vi "Dashboard Main.vi"() -> ()   [LabVIEW 2020]
uses:
  <vilib>/Utility/miscctls.llb/LVRectTypeDef.ctl
  <vilib>/Utility/miscctls.llb/LVRowAndColumnTypeDef.ctl
  <vilib>/event_ctls.llb/eventvkey.ctl
  <vilib>/Rock Robotics/WPI/DriverStation/WPI_DriverStationAllianceInfo.ctl
  b1c29fd4-b69e-4c47-bd92-218700034153.vi
  74f3c57e-8635-4bc1-b4f8-b214002a8360.vi
  a407d339-4daa-4cfa-a8dc-714c5dae658b.vi
  cd51690b-7cbe-44fb-a5f0-3232adb0ed53.vi
  a4e8d5d1-2ec3-4e81-be0b-60391cc68073.vi
  1b78be80-bab2-445d-a3e8-82f142a16380.vi
  9e807339-2903-4f51-8fcc-64b6a9381567.vi
  e75f20ac-3dfa-4544-8614-4803d6d17fbb.vi
  0137daef-9682-45ba-80b9-2d4fda8852b8.vi
  f6a63fab-964b-4051-8314-d4414a0a258c.vi
  90e0fe9d-42b1-4a72-a6c8-4b9d9b3a5a2a.vi
  f15e925d-3118-43e3-bf67-a1272bbf81dd.vi
  394886aa-4cdd-4740-8681-89e3e438764a.vi
  77a42c1f-99bf-4bb6-8218-45b49017f7dc.vi
  5abae45b-ab2b-4816-ba0c-2a0b218f6531.vi
  31f70c1d-3051-4c77-9544-a691198ba614.vi
  81d0db6a-d68a-45c3-b3b1-458879412541.vi
  7115eafd-0426-4044-a2c2-04b4175d5bfc.vi
  c235c188-eb56-46fb-93d3-e8acf396af31.vi
  115ba94a-0b26-47fa-ae73-5ec5bd9e502a.vi
  2422668c-951b-48e5-9bda-0f59c56d9c0d.vi
  7776664e-4af7-4b3d-b288-2266642a045e.vi
  ace04e1a-73bd-4435-b0d6-ff328b65c92e.vi
  6004ed5d-dfc4-4dad-95c1-8e371ea2b9cd.vi
  321ce103-7778-4bb1-9ecc-75a76fef05e9.vi
  d30e88cc-5e2b-4867-b271-53fc6d5cd4d7.vi
  fde90579-e212-4b8a-8145-a17c3e40bcbd.vi
  6c63589b-432e-4f9c-bacb-2063ed7bd576.vi
  b7dcf304-99f6-4f78-9d14-19aa8d9ea562.vi
  0480a820-69ef-45e6-a9f4-d7ff60c89e45.vi
  1c99237e-ea3d-4ecf-b7c2-61034db3ecd2.vi
  db817f79-2de4-4a0f-b1b3-d5e700c778e5.vi
  2e0df589-fb3d-4210-b682-2dd460d02044.vi
  7e0b6b61-ecd1-46e7-8bdd-33cde7d6a778.vi
  5b0403e5-003a-4f6e-89c5-e8c7c203eb26.vi
  f6dc994a-5b2f-4b9c-b35a-30746132b034.vi
  769dec14-fabd-470d-9aa2-970817a7097c.vi
  609bb688-569d-4125-8a50-26b015384e1e.vi
  de6d5f31-b9eb-4ae9-a598-d9fff82cebf9.vi
  24606ce8-9050-485a-8372-b08799457f70.vi
  c4f1d6a7-022d-437a-99da-c80f8ac5100c.vi
  c6e82f58-8c51-44a0-978c-3033ebe9f2a9.vi
  434a79fa-e0d6-40cd-a4b2-153fd9802099.vi
  16a0616d-4b31-4831-aeab-0be446d50f6a.vi
  0a8fe2ab-d060-4915-a9b5-d8978247e2b6.vi
  b1c29fd4-b69e-4c47-bd92-218700034153.vi/77c742ae-e671-49bb-a825-a6e8cebc9f63.vi
  74f3c57e-8635-4bc1-b4f8-b214002a8360.vi/77c742ae-e671-49bb-a825-a6e8cebc9f63.vi
  a407d339-4daa-4cfa-a8dc-714c5dae658b.vi/77c742ae-e671-49bb-a825-a6e8cebc9f63.vi
  cd51690b-7cbe-44fb-a5f0-3232adb0ed53.vi/77c742ae-e671-49bb-a825-a6e8cebc9f63.vi
  a4e8d5d1-2ec3-4e81-be0b-60391cc68073.vi/77c742ae-e671-49bb-a825-a6e8cebc9f63.vi
  1b78be80-bab2-445d-a3e8-82f142a16380.vi/77c742ae-e671-49bb-a825-a6e8cebc9f63.vi
  9e807339-2903-4f51-8fcc-64b6a9381567.vi/77c742ae-e671-49bb-a825-a6e8cebc9f63.vi
  e75f20ac-3dfa-4544-8614-4803d6d17fbb.vi/77c742ae-e671-49bb-a825-a6e8cebc9f63.vi
  0137daef-9682-45ba-80b9-2d4fda8852b8.vi/77c742ae-e671-49bb-a825-a6e8cebc9f63.vi
  f6a63fab-964b-4051-8314-d4414a0a258c.vi/77c742ae-e671-49bb-a825-a6e8cebc9f63.vi
  90e0fe9d-42b1-4a72-a6c8-4b9d9b3a5a2a.vi/77c742ae-e671-49bb-a825-a6e8cebc9f63.vi
  f15e925d-3118-43e3-bf67-a1272bbf81dd.vi/77c742ae-e671-49bb-a825-a6e8cebc9f63.vi
  394886aa-4cdd-4740-8681-89e3e438764a.vi/77c742ae-e671-49bb-a825-a6e8cebc9f63.vi
  77a42c1f-99bf-4bb6-8218-45b49017f7dc.vi/77c742ae-e671-49bb-a825-a6e8cebc9f63.vi
  5abae45b-ab2b-4816-ba0c-2a0b218f6531.vi/77c742ae-e671-49bb-a825-a6e8cebc9f63.vi
  31f70c1d-3051-4c77-9544-a691198ba614.vi/77c742ae-e671-49bb-a825-a6e8cebc9f63.vi
  81d0db6a-d68a-45c3-b3b1-458879412541.vi/77c742ae-e671-49bb-a825-a6e8cebc9f63.vi
  7115eafd-0426-4044-a2c2-04b4175d5bfc.vi/77c742ae-e671-49bb-a825-a6e8cebc9f63.vi
  c235c188-eb56-46fb-93d3-e8acf396af31.vi/77c742ae-e671-49bb-a825-a6e8cebc9f63.vi
  115ba94a-0b26-47fa-ae73-5ec5bd9e502a.vi/77c742ae-e671-49bb-a825-a6e8cebc9f63.vi
  2422668c-951b-48e5-9bda-0f59c56d9c0d.vi/77c742ae-e671-49bb-a825-a6e8cebc9f63.vi
  7776664e-4af7-4b3d-b288-2266642a045e.vi/77c742ae-e671-49bb-a825-a6e8cebc9f63.vi
  ace04e1a-73bd-4435-b0d6-ff328b65c92e.vi/77c742ae-e671-49bb-a825-a6e8cebc9f63.vi
  6004ed5d-dfc4-4dad-95c1-8e371ea2b9cd.vi/77c742ae-e671-49bb-a825-a6e8cebc9f63.vi
  321ce103-7778-4bb1-9ecc-75a76fef05e9.vi/77c742ae-e671-49bb-a825-a6e8cebc9f63.vi
  d30e88cc-5e2b-4867-b271-53fc6d5cd4d7.vi/77c742ae-e671-49bb-a825-a6e8cebc9f63.vi
  fde90579-e212-4b8a-8145-a17c3e40bcbd.vi/77c742ae-e671-49bb-a825-a6e8cebc9f63.vi
  6c63589b-432e-4f9c-bacb-2063ed7bd576.vi/77c742ae-e671-49bb-a825-a6e8cebc9f63.vi
  b7dcf304-99f6-4f78-9d14-19aa8d9ea562.vi/77c742ae-e671-49bb-a825-a6e8cebc9f63.vi
  0480a820-69ef-45e6-a9f4-d7ff60c89e45.vi/77c742ae-e671-49bb-a825-a6e8cebc9f63.vi
  1c99237e-ea3d-4ecf-b7c2-61034db3ecd2.vi/77c742ae-e671-49bb-a825-a6e8cebc9f63.vi
  db817f79-2de4-4a0f-b1b3-d5e700c778e5.vi/77c742ae-e671-49bb-a825-a6e8cebc9f63.vi
  2e0df589-fb3d-4210-b682-2dd460d02044.vi/77c742ae-e671-49bb-a825-a6e8cebc9f63.vi
  7e0b6b61-ecd1-46e7-8bdd-33cde7d6a778.vi/77c742ae-e671-49bb-a825-a6e8cebc9f63.vi
  5b0403e5-003a-4f6e-89c5-e8c7c203eb26.vi/77c742ae-e671-49bb-a825-a6e8cebc9f63.vi
  f6dc994a-5b2f-4b9c-b35a-30746132b034.vi/77c742ae-e671-49bb-a825-a6e8cebc9f63.vi
  769dec14-fabd-470d-9aa2-970817a7097c.vi/77c742ae-e671-49bb-a825-a6e8cebc9f63.vi
  609bb688-569d-4125-8a50-26b015384e1e.vi/77c742ae-e671-49bb-a825-a6e8cebc9f63.vi
  de6d5f31-b9eb-4ae9-a598-d9fff82cebf9.vi/77c742ae-e671-49bb-a825-a6e8cebc9f63.vi
  24606ce8-9050-485a-8372-b08799457f70.vi/77c742ae-e671-49bb-a825-a6e8cebc9f63.vi
  c4f1d6a7-022d-437a-99da-c80f8ac5100c.vi/77c742ae-e671-49bb-a825-a6e8cebc9f63.vi
  c6e82f58-8c51-44a0-978c-3033ebe9f2a9.vi/77c742ae-e671-49bb-a825-a6e8cebc9f63.vi
  434a79fa-e0d6-40cd-a4b2-153fd9802099.vi/77c742ae-e671-49bb-a825-a6e8cebc9f63.vi
  16a0616d-4b31-4831-aeab-0be446d50f6a.vi/77c742ae-e671-49bb-a825-a6e8cebc9f63.vi
  0a8fe2ab-d060-4915-a9b5-d8978247e2b6.vi/77c742ae-e671-49bb-a825-a6e8cebc9f63.vi
  <vilib>/Utility/xml.llb/Read From XML File(array).vi
  <vilib>/Utility/xml.llb/Write to XML File(string).vi
  <vilib>/Rock Robotics/Network Tables/NT Read Boolean.vi
  <vilib>/Rock Robotics/Network Tables/NT Write Number.vi
  <vilib>/Rock Robotics/Network Tables/NT Read Numeric Array.vi
  <vilib>/Rock Robotics/Network Tables/NT Write Boolean.vi
  <vilib>/Rock Robotics/Network Tables/NT Read String Array.vi
  <vilib>/Rock Robotics/Network Tables/NT Read Boolean Array.vi
  <vilib>/Rock Robotics/Network Tables/NT Write String.vi
  <vilib>/Rock Robotics/Network Tables/NT Write Numeric Array.vi
  <vilib>/Rock Robotics/WPI/Dashboard/WPI_DashboardLogging Global.vi
  <vilib>/Rock Robotics/Network Tables/NT Write String Array.vi
  <vilib>/vision/NI_Vision_Development_Module.lvlib
panel:
  in  "TCP":refnum<k5>
  out "Image Message":string="Timeout in Camera Communications"
  in  "Dashboard Tab":T1(tab)=enum."Setup/Auto"
  in  "CheckList":i32(listbox)
  in  "Enable_Streaming_GUI":bool=TRUE
  out "Robot_Profile_GUI":string
  out "Auto_Playbook_GUI":string
  in  "Driver Profile (1)":u16(ring) items=["N/A"]
  in  "Camera Name":string(combo)="limelight"
  in  "Camera Settings":T2={"Frame Rate"=20, "Compression"=60, "Size"=1, "DB Camera Config"=FALSE} {"Size" items=["640x480", "320x240", "160x120"]}
  in  "Select Autonomous Play":u16(ring) items=["N/A"]
  out "Master_Caution_GUI_0":bool caption="Mode_Butterfly"
  out "Robot_is_Autonomous_GUI_0":bool caption="Mode_Butterfly"
  out "Robot_Code_Version_GUI":string
  out "Auto_Suffix_GUI":string
  in  "Refresh_Auto_Play_List_GUI":bool
  in  "Auto_Delay_GUI":dbl format="%.1f"
  in  "Manual_Start_X":dbl=324.0 format="%.1f"
  out "Robot_X":dbl format="%.1f"
  out "Robot_Y":dbl format="%.1f"
  in  "Manual_Start_Y":dbl=50.0 format="%.1f"
  out "Robot_H_GUI":dbl format="%.1f"
  in  "Manual_Start_H":dbl format="%.1f"
  out "Range_To_Target_GUI":dbl format="%.1f"
  in  "Field Map":u16(ring) items=["N/A"]
  in  "Push_Robot_Start_GUI":bool
  in  "Export_Robot_Pose":bool
  in  "Clear_Robot_Pose_Display":bool
  in  "Dock_Dashboard":bool
  in  "Force_Human_Control_GUI":bool
  in  "Auto_Test_Mode_GUI":bool
  out "Angle_To_Target_GUI":dbl format="%.1f"
  out "Turret_H_GUI":dbl format="%.1f"
  in  "Disable_Fusion_While_Autonomous":bool
  in  "Disable_Fusion_While_Disabled":bool=TRUE
  in  "New_HUB_Height_Offset_GUI":dbl min=-99.0 max=99.0 step=1.0 format="%.1f"
  out "Current_HUB_Height_Offset_GUI":dbl format="%.1f"
  in  "Apply_New_HUB_Height_Offset_GUI":bool
  out "Robot Pose 1":cluster{dbl[], dbl[]}[](graph)
  out "Help Graphic":T3(plugin-control)
  out "Master_State_1_Indicator":bool
  out "Master_State_0_Indicator":bool
  out "Shooter_State_3_Indicator":bool
  out "Shooter_State_2_Indicator":bool
  out "Shooter_State_1_Indicator":bool
  out "Kicker_Overheating_GUI":bool
  out "Robot Pose 2":cluster{dbl[], dbl[]}[](graph)
  out "Shooter_Upper_Overheating_GUI":bool
  out "Intake_Motor_Failure_Left_GUI":bool
  out "Vision_Fault_GUI":bool
  out "Pressure_Leak_GUI":bool
  in  "Master_Safety_Override_1":bool
  in  "Manipulator_Help":bool
  in  "Driver_Help":bool
  in  "Error_Help":bool
  out "No_Secondary_Camera":bool
  out "Swerve_Shifter_Failure":bool
  out "Electrical_Fault_GUI":bool
  out "Diverting_Power_GUI":bool
  out "CAN_Bus_Fault_GUI":bool
  out "IMU_Failure_GUI":bool
  out "Robot_is_Autonomous_GUI_1":bool caption="Mode_Butterfly"
  out "LL_Valid":bool caption="Mode_Butterfly"
  out "Current_Balls_GUI":i32 format="%#.0f"
  out "Intake_Motor_Failure_Right_GUI":bool
  out "CARGO_Ret_Left":bool
  out "CARGO_Ret_Right":bool
  out "Intake_Intaking_GUI":bool caption="Mode_Butterfly"
  out "Shooter_Lower_Overheating_GUI":bool
  out "Auto_Error_GUI":bool
  in  "Clear_Errors_GUI":bool
  out "Swerve_Azimuth_Fault":bool
  out "Pressure_Transducer_GUI":dbl(slide) scale=0.0..115.0
  out "Pressure_Vent_GUI":bool
  out "Swerve_Overheating":bool
  out "Compressor_On_GUI":bool
  out "HUB_Ret_Right":bool
  out "HUB_Ret_Left":bool
  in  "Right":bool
  in  "Reticule":T4(ring)
  in  "Save":bool
  in  "Up":bool
  in  "Down":bool
  in  "Left":bool
  out "Master_Caution_GUI_1":bool caption="Mode_Butterfly"
  out "Battery_Critical_GUI":bool
  out "Battery_Voltage_GUI":dbl(slide) scale=11.0..13.0
  out "Field_Oriented_GUI":bool caption="Mode_Butterfly"
  out "Slow_Loop":bool
  out "Arm_Climber":bool
  out "Combined Camera Feed":T3(plugin-control)
  out "Pointed_At_Target_GUI":bool caption="Mode_Butterfly"
  out "Shooter_Ready_GUI":bool caption="Mode_Butterfly"
  out "Shooter_Firing_GUI":bool caption="Mode_Butterfly"
  out "Shooter_Spinning_GUI":bool caption="Mode_Butterfly"
  out "Climber_Climbing_GUI":bool caption="Mode_Butterfly"
  out "Range_To_Target_GUI_Small":dbl
  out "Angle_To_Target_GUI_Small":dbl
  out "Shooter_State_0_Indicator":bool
  out "Shooter_State_4_Indicator":bool
  in  "Auto_Indexing_Override_GUI":bool
  in  "Auto_Target_Override_GUI":bool
  in  "Camera_Override_GUI":bool
  in  "Field_Oriented_Override_GUI":bool
  in  "Apply_Radial_Firing_Delay_GUI":bool
  out "Selected_Radial_Firing_Delay_GUI":dbl format="%.2f"
  in  "New_Radial_Firing_Delay_GUI":dbl min=0.0 max=5.0 step=0.1 format="%.2f"
  out "Kicker_Temperature_GUI":dbl
  out "Kicker_Speed_GUI":dbl
  in  "New_Shooter_Setpoint_Angle_GUI":dbl=11.0 min=11.0 max=36.0 step=1.0 format="%.2f"
  out "Selected_Shooter_Setpoint_Angle_Value_GUI":dbl format="%.2f"
  in  "Home_Cowl_GUI":bool
  out "Indexer_Beam_Break_GUI":bool caption="Mode_Butterfly"
  out "Cowl_Limit_A_GUI":bool caption="Mode_Butterfly"
  out "Turret_Limit_B_GUI":bool caption="Mode_Butterfly"
  out "Turret_Limit_A_GUI":bool caption="Mode_Butterfly"
  out "Turret_Angle_GUI":dbl format="%.1f"
  out "Cowl_Angle_GUI":dbl format="%.2f"
  out "Shooter_Upper_Temperature_GUI":dbl
  out "Swerve_3_Drive_Velocity":dbl format="%.1f"
  out "Swerve_3_Azimuth_Position":dbl format="%.1f"
  out "Swerve_3_Drive_Temperature":dbl
  out "Swerve_0_Drive_Temperature":dbl
  out "Camera Perf":string
  out "Control_Loop_Time_GUI":u32
  in  "Calibrate_Wheels_GUI":bool
  in  "Home_Wheels_GUI":bool
  out "Swerve_0_Azimuth_Position":dbl format="%.1f"
  out "Swerve_0_Drive_Velocity":dbl format="%.1f"
  out "Swerve_1_Drive_Velocity":dbl format="%.1f"
  out "Swerve_1_Azimuth_Position":dbl format="%.1f"
  out "Swerve_1_Drive_Temperature":dbl
  out "Swerve_2_Drive_Velocity":dbl format="%.1f"
  out "Swerve_2_Azimuth_Position":dbl format="%.1f"
  out "Swerve_2_Drive_Temperature":dbl
  in  "Arm_Calibrate_Wheels_GUI":bool
  out "Master_Caution_GUI_2":bool caption="Mode_Butterfly"
  out "Shooter_Lower_Temperature_GUI":dbl
  out "Shooter_Upper_Speed_GUI":dbl
  in  "New_Shooter_Setpoint_Speed_GUI":dbl=2000.0 min=0.0 max=5700.0 step=100.0 format="%#.0f"
  in  "Actuator Testing":u16(ring) items=["N/A"]
  in  "Test_Actuator_Value_GUI":dbl step=0.1 format="%.2f"
  in  "Calibrate_Joysticks_GUI":bool
  in  "Arm_Calibrate_Joysticks":bool
  out "Robot_is_Autonomous_GUI_2":bool caption="Mode_Butterfly"
  in  "Test_Actuator_Period_GUI":dbl min=0.0 step=1.0 format="%.2f"
  out "Pose_Loop_Time_GUI":u32
  in  "Mute_Audible_Warnings":bool
  out "Combined Error String":string
  out "Swerve_0_Shifter_State":string
  out "Swerve_1_Shifter_State":string
  out "Swerve_3_Shifter_State":string
  out "Swerve_2_Shifter_State":string
  out "Swerve_Azimuth_Fault_Array":bool[](array[boolean])
  out "Selected_Shooter_Setpoint_Speed_Value_GUI":dbl
  in  "Apply_New_Shooter_Setpoint_GUI":bool
  in  "Selected_Shooter_Setpoint_Index":u16(ring) items=["N/A"]
  in  "Super_Test_Mode_GUI":bool
  out "Current_Driver_Profile_Setpoints_GUI":T5={"Strafe Deadband"=0.08, "Strafe Scaling"=2.0, "Strafe Maximum"=0.5, "Rotation Deadband"=0.15, "Rotation Scaling"=2.5, "Rotation Maximum"=0.5} {"Rotation Maximum" min=0.3 max=1.0 scale=0.3..1.0; "Rotation Scaling" min=1.0 max=4.0 scale=1.0..4.0; "Rotation Deadband" min=0.0 max=0.25 scale=0.0..0.25; "Strafe Maximum" min=0.3 max=1.0 scale=0.3..1.0; "Strafe Scaling" min=1.0 max=4.0 scale=1.0..4.0; "Strafe Deadband" min=0.0 max=0.25 scale=0.0..0.25}
  in  "New_Driver_Profile_Setpoints_GUI":T6={"Strafe Deadband"=0.08, "Strafe Scaling"=2.0, "Strafe Max"=0.5, "Rotate Deadband"=0.15, "Rotate Scaling"=2.5, "Rotate Max"=0.5} {"Rotate Max" min=0.3 max=1.0 format="%.2g"; "Rotate Scaling" min=1.0 max=4.0 format="%.2g"; "Rotate Deadband" min=0.0 max=0.25 format="%.2g"; "Strafe Max" min=0.3 max=1.0 format="%.2g"; "Strafe Scaling" min=1.0 max=4.0 format="%.2g"; "Strafe Deadband" min=0.0 max=0.25 format="%.2g"}
  in  "Apply_Driver_Profile_Setpoints_GUI":bool
  out "Current_Driver_Profile_GUI":string
  in  "Home_Turret_GUI":bool
  out "Shooter_Lower_Speed_GUI":dbl
  out "Tower_Beam_Break_GUI":bool caption="Mode_Butterfly"
  out "Color_Sensor_Reading_GUI":string
  out "Selected_Shooter_Setpoint_Ratio_Value_GUI":dbl format="%.2f"
  in  "New_Shooter_Setpoint_Ratio_GUI":dbl=1.0 min=0.0 max=3.0 step=0.1 format="%.2f"
  out "Climber_Active_Arm_Position_GUI":dbl format="%.1f"
  in  "Free_Tuning_Variable_GUI":dbl min=0.0 step=1.0 format="%.3f"
  in  "Apply_Firing_Delay_GUI":bool
  out "Selected_Firing_Delay_GUI":dbl format="%.2f"
  in  "New_Firing_Delay_GUI":dbl min=0.0 max=5.0 step=0.1 format="%.2f"
  out "Selected_Shooter_Setpoint_Turret_Value_GUI":dbl format="%.1f"
  in  "New_Shooter_Setpoint_Turret_GUI":dbl min=-145.0 max=145.0 step=1.0 format="%.1f"
  in  "Targeting_Override_GUI":dbl(slide)=1.0 min=0.0 max=2.0 step=1.0 scale=0.0..2.0
  out "Audible_Warnings_Enabled_GUI":bool
  out "Legal_Drivers_GUI":string[](array[string])
  out "Swerve_Shifter_Failure_Array":bool[](array[boolean])
  out "Swerve_Overheating_Array":bool[](array[boolean])
  out "NT Connection":bool
  out "Mode":T7(ring)=enum."Auto Disabled"
  out "Progress":T8 {"Test Progress" scale=0.0..100.0}
  out "Cmd Status":string
  in  "Execute Command":bool
  in  "Command Params":string[][](table)
  in  "Command Selection":i32(listbox)
  out "Tree":string(tree)
  out "Background":bool
  # "2022 Dashboard v4.2-stable"
  # "Robot Profile"
  # "Robot X Position (in)"
  # "Robot Y Position (in)"
  # "Auto Play Suffix"
  # "Auto Delay (s)"
  # "X (in)"
  # "Robot Heading (deg)"
  # "Autonomous Playbook Entry"
  # "Auto Test\nMode"
  # "Force\nHuman"
  # "Turret Heading (deg)"
  # "Y (in)"
  # "Range to Target (in)"
  # "H (deg)"
  # "Angle to Target (deg)"
  # "Undock Dashboard"
  # "Yes Camera Streaming"
  # "Stop Fusion While Auto"
  # "Stop Fusion While Disabled"
  # "+X"
  # "+Y"
  # "HUB Height Offset (in)"
  # "MASTER\nSTATES"
  # "OVERRIDES"
  # "Camera Override (3)"
  # "Robot-Oriented Drive Controls"
  # "BALLS"
  # "SHOOTER\nSTATES"
  # "Manual Indexing (4)"
  # "Lock Turret to Center"
  # "(2)"
  # "SAFETY\nOVERRIDE"
  # "11"
  # "13"
  # "0"
  # "115"
  # "Drivebase Subsytem"
  # "Shooter and Turret Subsystems"
  # "Driver Profile Configuration"
  # "Shooter Setpoints"
  # "Control"
  # "Pose"
  # "Module 1"
  # "Module 0"
  # "Kicker"
  # "Latency\n(ms)"
  # "Lower"
  # "Upper"
  # "Azimuth (deg)"
  # "Speed  (rpm)"
  # "Speed (rpm)"
  # "Temp (C)"
  # "Temp (C)"
  # "Super Test Mode"
  # "Variable (bleh)"
  # "Velocity (ft/s)"
  # "Speed Ratio"
  # "Cowl"
  # "Turret"
  # "Shifter State"
  # "Angle (deg)"
  # "Angle (deg)"
  # "Module 2"
  # "Module 3"
  # "Target Selection"
  # "Limit Switches"
  # "Azimuth (deg)"
  # "Turret (deg)"
  # "Temp (C)"
  # "Calibrate Turret"
  # "Calibrate Cowl"
  # "HUB"
  # "AUTO"
  # "HANG"
  # "Velocity (ft/s)"
  # "Shifter State"
  # "Amplitude"
  # "Period (s)"
  # "Tangential Shooting Delay (s)"
  # "Calibrate Wheels"
  # "Ball Handling Subsystem"
  # "Climber Subsystem"
  # "Radial Shooting Delay (s)"
  # "Beam Breaks"
  # "Active Arms"
  # "Calibrate Joysticks"
  # "Color"
  # "Position (in)"
  # "0"
  # "0.25"
  # "1"
  # "4"
  # "0.3"
  # "1"
  # "0"
  # "0.25"
  # "1"
  # "4"
  # "0.3"
  # "1"
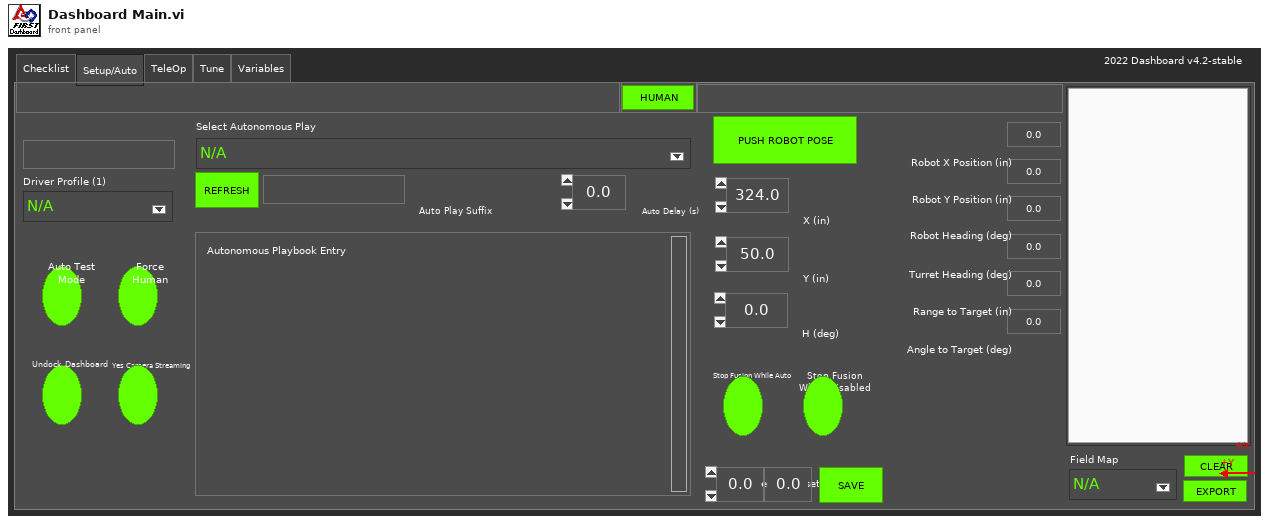
[diagram p1: front panel]
types:
  T1 = enum32{"Checklist", "Setup/Auto", "TeleOp", "Tune", "NT", "Test", "Commands", "Variables"}
  T2 = cluster{"Frame Rate":i32, "Compression":i32, "Size":u16, "DB Camera Config":bool}
  T3 = typedef "IMAQ Image.ctl" = refnum<image>
  T4 = enum16{"HUB Left Reticule", "HUB Right Reticule", "CARGO Left Reticule", "CARGO Right Reticule"}
  T5 = cluster{"Strafe Deadband":dbl, "Strafe Scaling":dbl, "Strafe Maximum":dbl, "Rotation Deadband":dbl, "Rotation Scaling":dbl, "Rotation Maximum":dbl}
  T6 = cluster{"Strafe Deadband":dbl, "Strafe Scaling":dbl, "Strafe Max":dbl, "Rotate Deadband":dbl, "Rotate Scaling":dbl, "Rotate Max":dbl}
  T7 = enum8{"Tele-Op Disabled", "Tele-Op Enabled", "Auto Disabled", "Auto Enabled", "Test Disabled", "Test Enabled", "Disconnected", "No Code", "E-Stop"}
  T8 = cluster{"Test Progress":u8, "Test Progress Text":string}
  T9 = cluster{"Save Path":path, "Interval (s)":dbl, "Keep":i32}
  T10 = enum32{"Drive", "Camera", "Basic", "Custom", "Test", "Commands", "Checklist", "Variables"}
  T11 = cluster{"IDs":cluster{"RPC field ID":u16, "Unique ID":u16}, "String":string}
  T12 = typedef "Image Type" = u32
  T13 = cluster{"HUB_Ret_Left":refnum<vi>, "HUB_Ret_Right":refnum<vi>, "CARGO_Ret_Left":refnum<vi>, "CARGO_Ret_Right":refnum<vi>}
  T14 = cluster{"Camera Name":string, string, "Saved DB Images Info":cluster{"Save Path":path, "Interval (s)":dbl, "Keep":i32}}
  T15 = typedef "WPI_DriverStationAllianceInfo.ctl" = enum16{"Red", "Blue", "Invalid"}
  T16 = enum8{"Enabled", "Disabled", "Disabled and Grayed Out"}
  T17 = cluster{"Error Strings":string, "Disable Counts":cluster{u16, u16}, "Rail Faults":cluster{u16, u16, u16}, "Robot IP":string, "DB Mode":u8, "Event Info":cluster{"Name":string, "Type":u8, "Number":u16, "Replay":u8}}
  T18 = cluster{"Storage":cluster{"Disk Free":u64, "RAM Block":u32, "RAM free":u32}, "CPU Utilization":cluster{"CPU % ISR":sgl, "CPU % Time Crit":sgl, "CPU % Timed Str":sgl, "CPU % High":sgl, "CPU % Above":sgl, "CPU % Normal":sgl, "CPU % Low":sgl}, "CAN":cluster{"% Bus Utilization":sgl, "Bus Off Cnt":u32, "TX_FIFO Full Cnt":u32, "Receive Error Cnt":u8, "Transmit Error Cnt":u8}, "HID":cluster{"HID Outputs":u32, "Rumble Low":u16, "Rumble High":u16}[]}
  T19 = cluster{"Status bits":cluster{"Test Mode":bool, "Autonomous":bool, "Enabled":bool, "Code Start":bool, "Brownout":bool, "Reserved 2":bool, "Reserved 3":bool, "E-Stop":bool}, "Code Trace":cluster{"Disabled":bool, "TeleOp":bool, "Auto":bool, "Test":bool}, "Controller Type":enum16{"unknown", "cRIO", "roboRio"}, "Code?":enum16{"unknown", "noCode", "code"}, "Battery V":dbl}
  T20 = cluster{"Control Bits":cluster{"TestMode":bool, "Autonomous":bool, "Enabled":bool, "FMS Present":bool, bool, bool, bool, "E-Stop":bool}, "Team Station ":u8, "Countdown":sgl, "Joystick Values":cluster{"Axes":dbl[], "Buttons":bool[], "POVs":i16[]}[]}
  T21 = typedef "imagedata.ctl" = cluster{"image type":i32, "image depth":i32, "image":u8[], "mask":u8[], "colors":u32[], "Rectangle":cluster{"left":i16, "top":i16, "right":i16, "bottom":i16}}
  T22 = cluster{"Boolean":bool, "Numeric Text.Text Colors:Text Color":u32}
  T23 = cluster{"Numeric Array[0]":dbl, "Numeric Array[1]":dbl, "Numeric Array[2]":dbl, "Numeric Array[3]":dbl, "Numeric Array[4]":dbl, "Numeric Array[5]":dbl}
  T24 = cluster{"Operation":enum16{"Update", "Clear"}, "Color Box":u32}[]
  T25 = typedef "eventvkey.ctl" = enum16{"ASCII", "Enter", "Return", "Shift", "Ctrl", "Alt", "Cmd", "Opt", "Caps", "NumLock", "Clear", "Break", "Up", "Down", "Left", "Right", "Insert", "Delete", "Home", "End", "PageUp", "PageDown", "Escape", "Help", "Pause", "ScrollLock", "F1", "F2", "F3", "F4", "F5", "F6", "F7", "F8", "F9", "F10", "F11", "F12", "F13", "F14", "F15", "F16", "F17", "F18", "F19", "F20", "F21", "F22", "F23", "F24", "Play", "VolumeUp", "VolumeDown", "Mute", "Two Byte Char"}
  T26 = cluster{"Operation":enum16{"Update", "Clear"}, "Color Box":u32}
  T27 = typedef "LVRowAndColumnTypeDef.ctl" = cluster{"Row":i32, "Column":i32}
  T28 = cluster{"Shift":bool, "Ctrl":bool, "Alt":bool, "Cmd":bool, "Opt":bool}
  T29 = cluster{string, "Intake_Motor_Failure_Left_GUI":bool, dbl}
  T30 = cluster{string, "Swerve_Shifter_Failure":bool, dbl}
  T31 = cluster{string, "Master_Safety_Override_1":bool, dbl}
  T32 = cluster{string, "Swerve_Azimuth_Fault":bool, dbl}
  T33 = cluster{string, "Arm_Calibrate_Wheels_GUI":bool, dbl}
  T34 = cluster{string, "Intake_Motor_Failure_Right_GUI":bool, dbl}
  T35 = cluster{string, "Electrical_Fault_GUI":bool, dbl}
  T36 = cluster{string, "Arm_Calibrate_Joysticks":bool, dbl}
  T37 = typedef "LVRectTypeDef.ctl" = cluster{"Left":i16, "Top":i16, "Right":i16, "Bottom":i16}
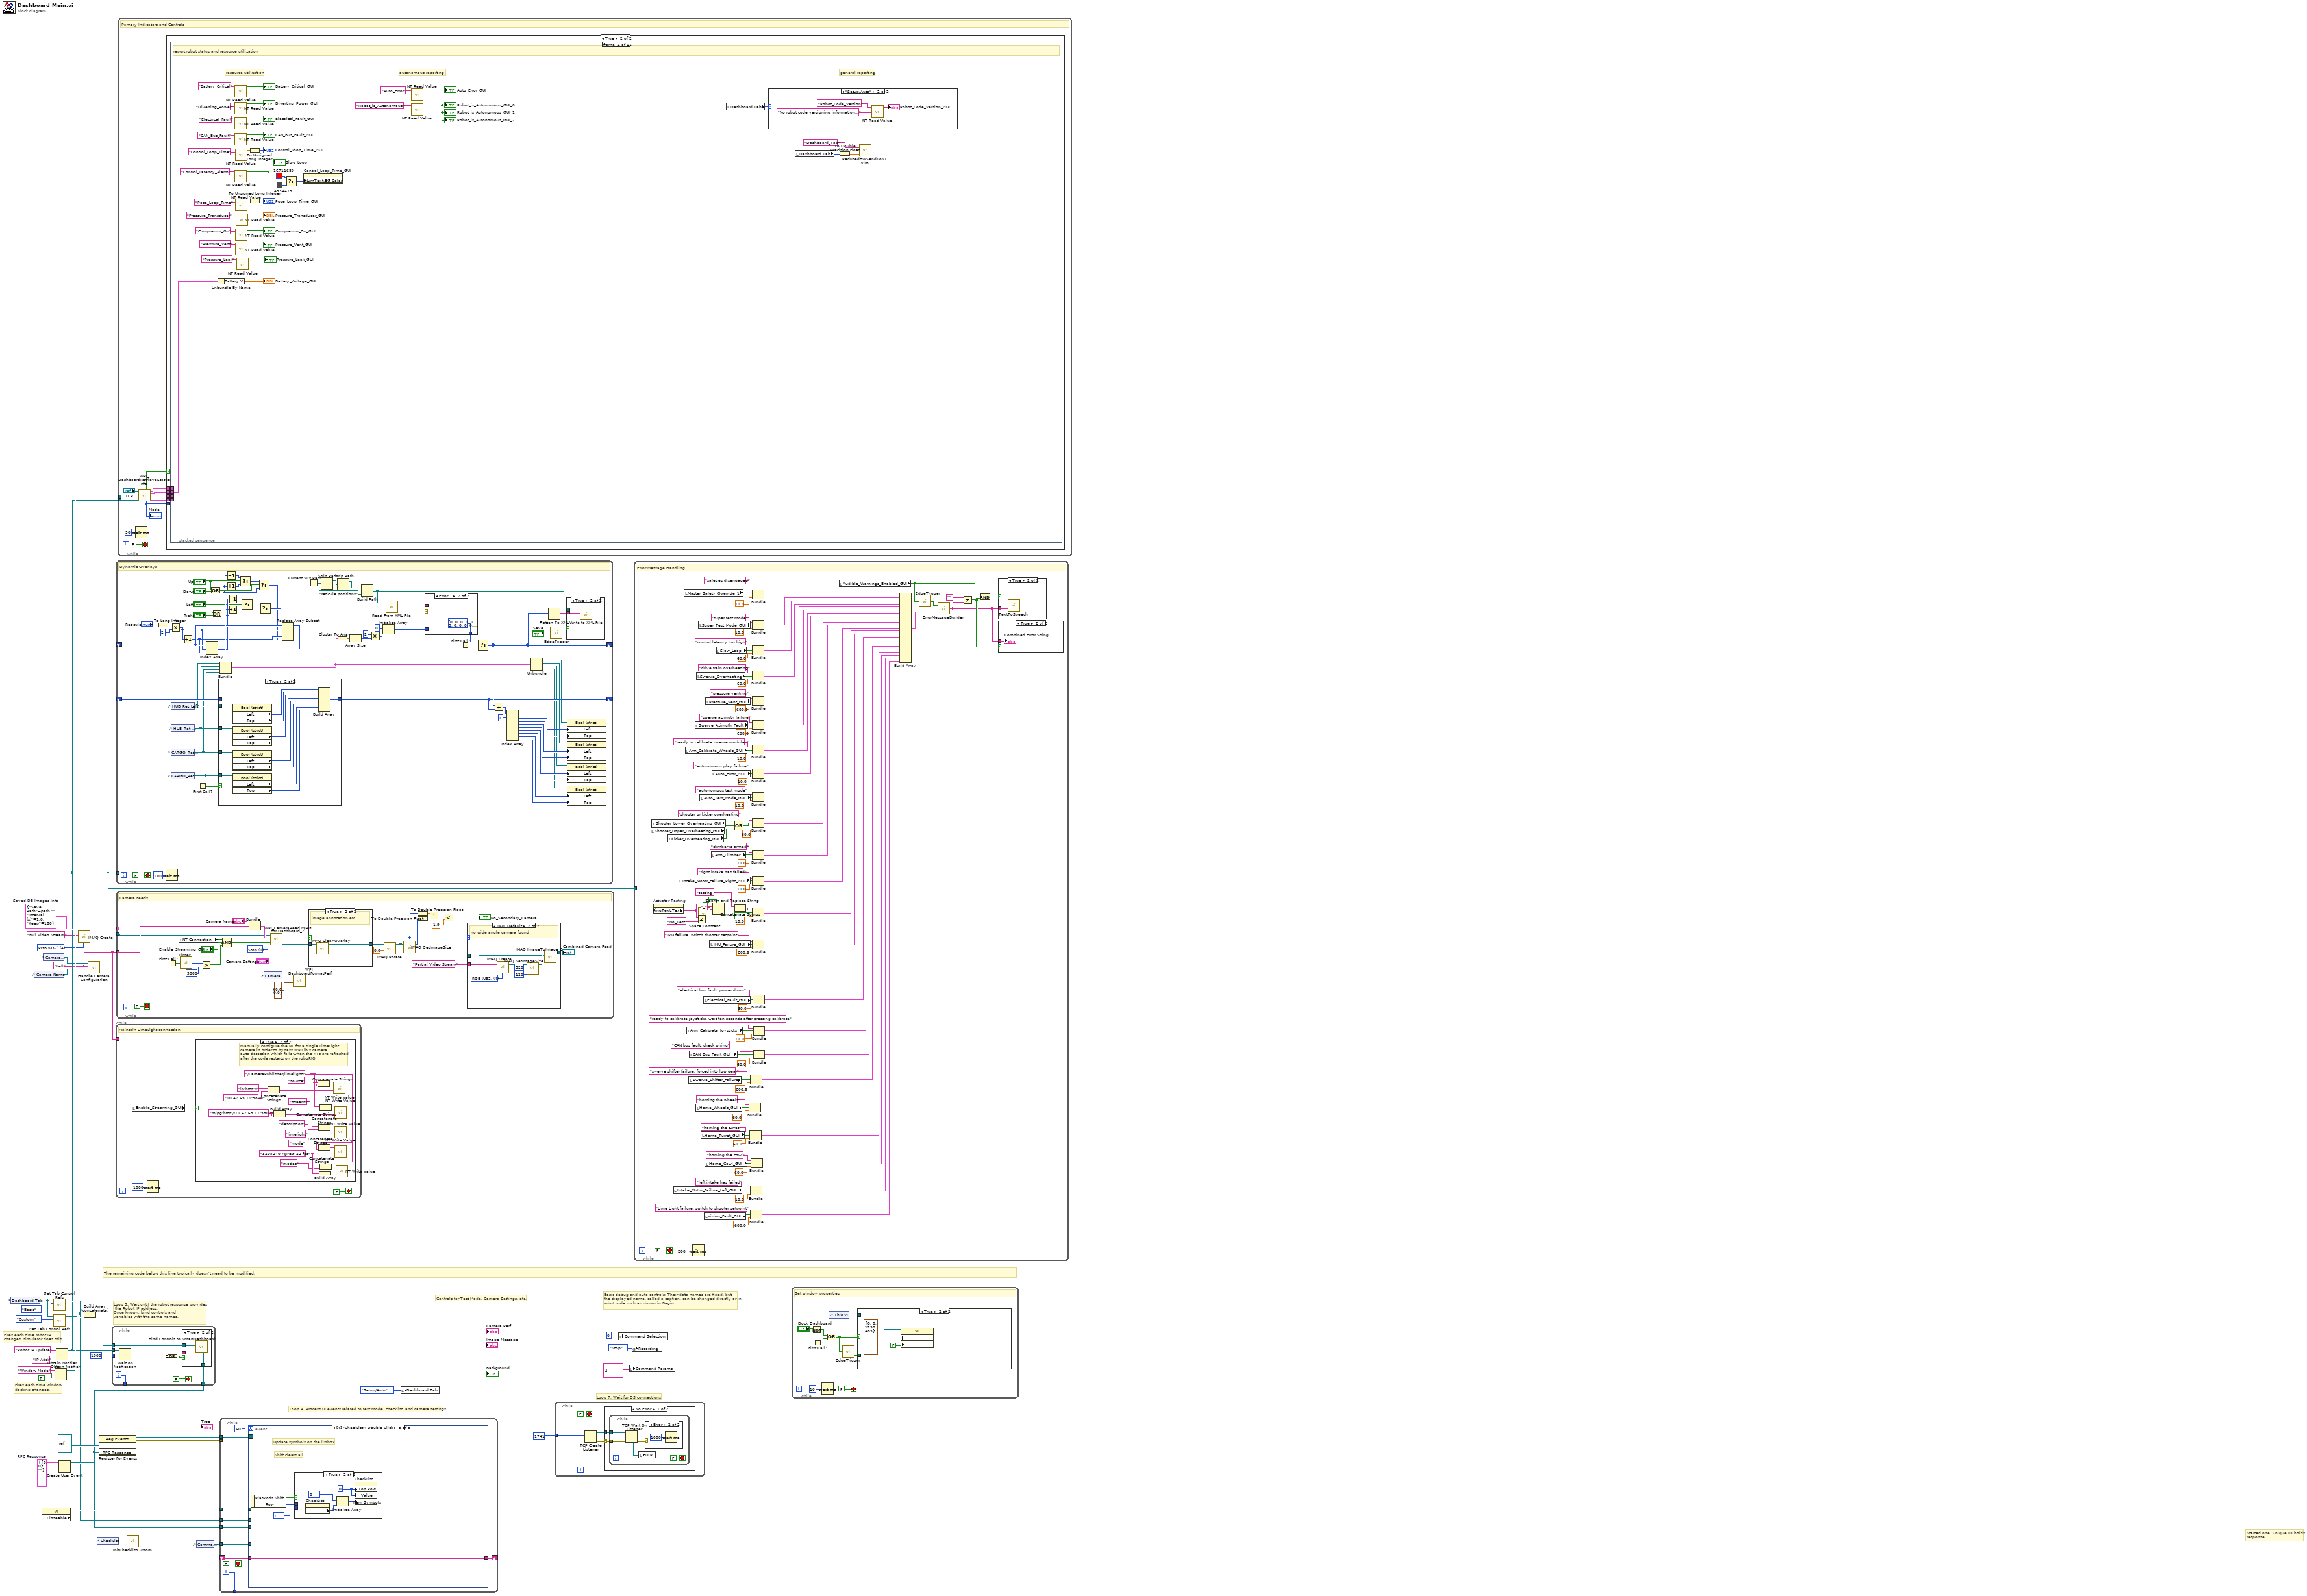
[diagram p0: block diagram]
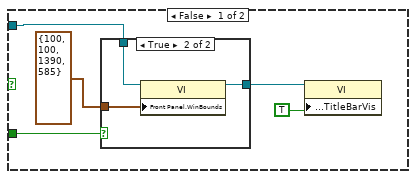
[diagram p3: hidden frame]
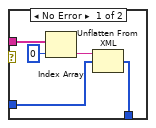
[diagram p7: hidden frame]
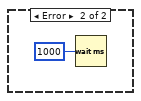
[diagram p11: hidden frame]
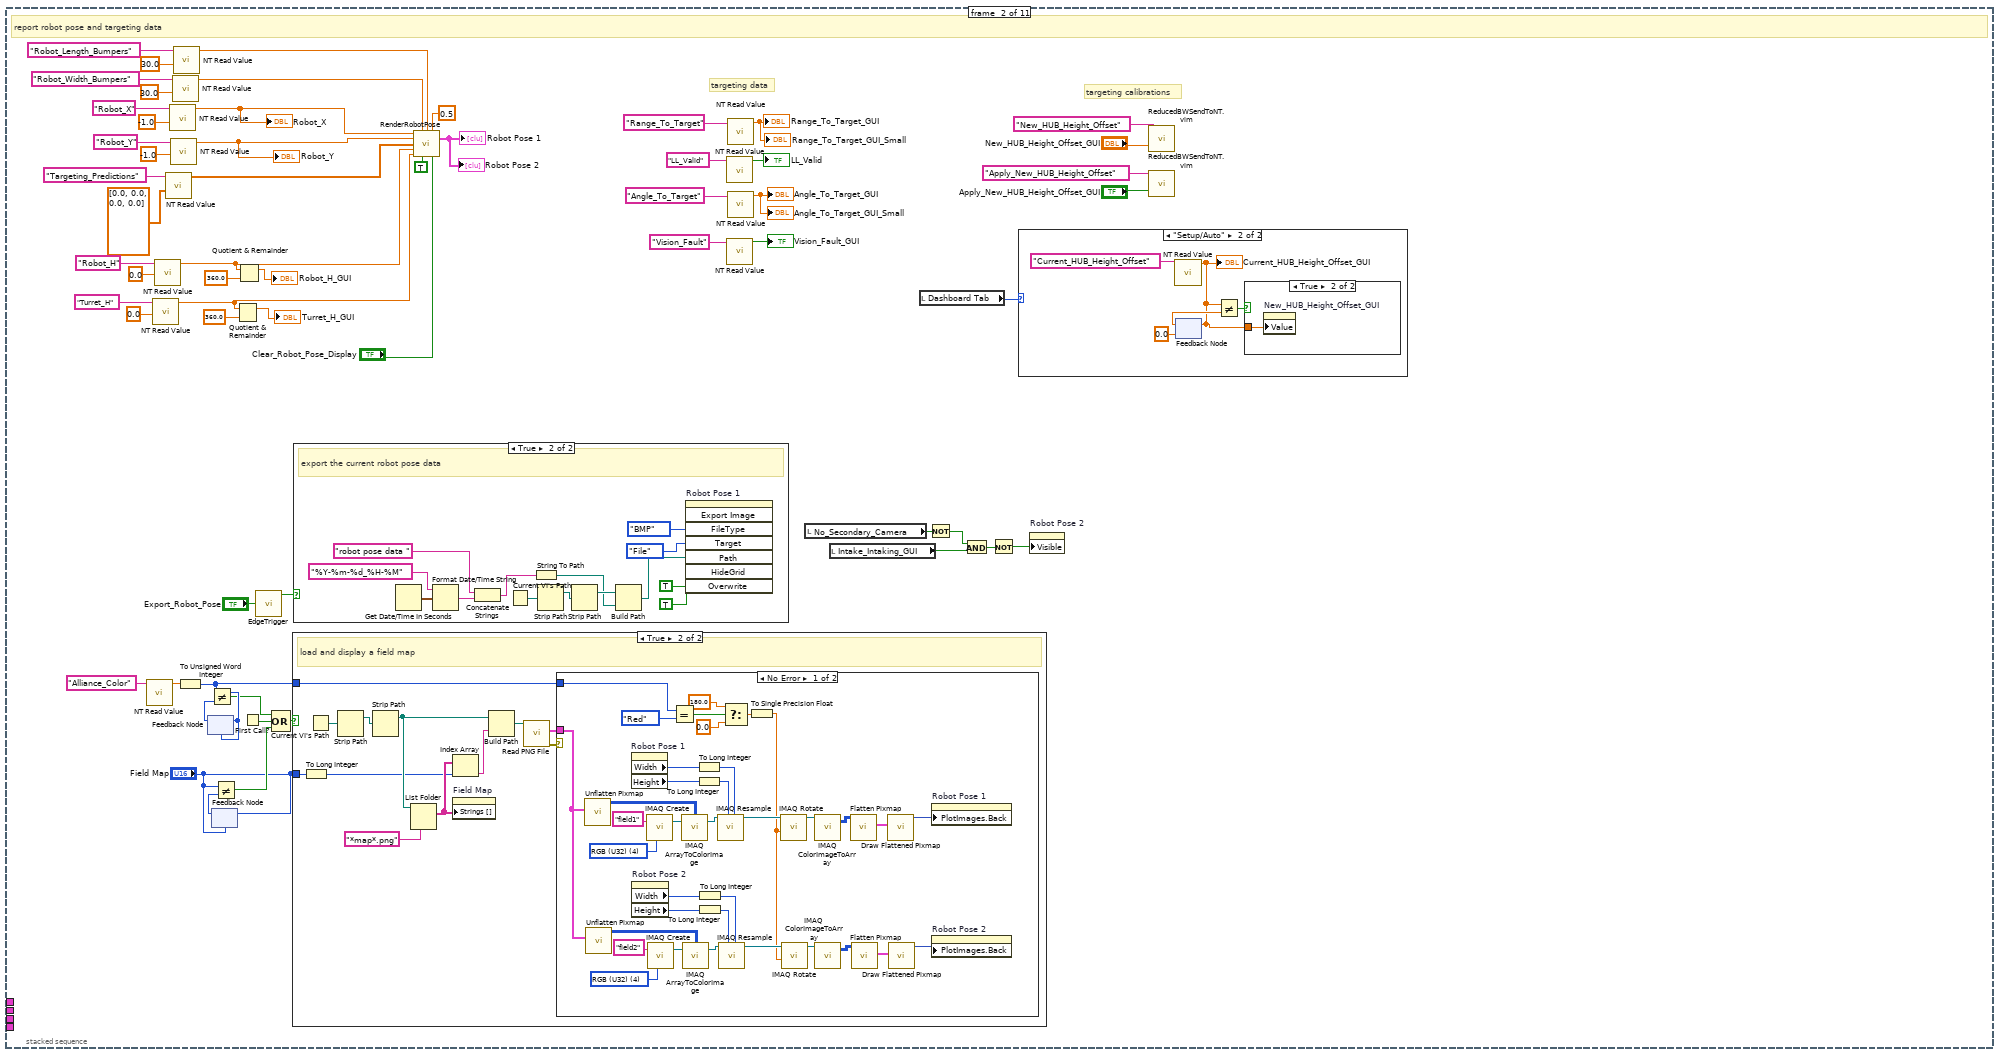
[diagram p14: hidden frame]
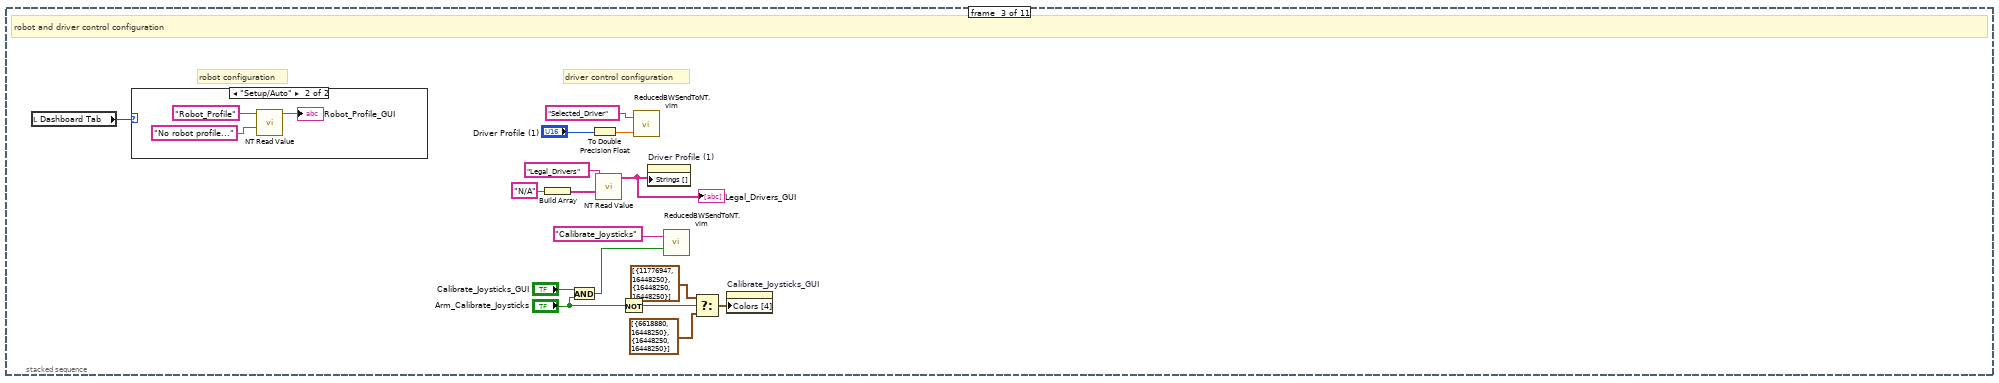
[diagram p20: hidden frame]
diagram:
  w9 = T9 {"Save Path"=path "", "Interval (s)"=1.0, "Keep"=180}  # Saved DB Images Info
  w1 = "Left"
  w17 = T11 {"IDs"={"RPC field ID"=0, "Unique ID"=0}, "String"=""}  # RPC Response
  w4 = T12 4 items=["Grayscale (U8)", "Grayscale (I16)", "Grayscale (SGL)", "Complex (CSG)", "RGB (U32)", "HSL (U32)", "RGB (U64)"] ("Image Type")
  # "Started one, Unique ID holds\nresponse"
  # "Loop 7. Wait for DS connections"
  # "Basic debug and auto controls: Their data names are fixed, but\nthe displayed name, called a caption, can be changed directly or in\nrobot code such as shown in Begin."
  # "Controls for Test Mode, Camera Settings, etc."
  # "Fires each time robot IP\nchanges, simulator does this"
  # "Fires each time window\ndocking changes."
  # "The remaining code below this line typically doesn't need to be modified."
  # "Loop 4. Process UI events related to test mode, checklist, and camera settings"
  # "Loop 3. Wait until the robot response provides\n the Robot IP address.\nOnce known, bind controls and\nvariables with the same names."
  n1 = control-ref of="Dashboard Tab"() -> (w23:refnum<vi>)
  n2 = control-ref of="Camera Name"() -> (w6:refnum<vi>)
  n3 = property class="VI" props=["Front Panel.Closeable"]() -> (reference out=w24:refnum<vi>)  [unwired: 2 in, 2 out]
  n4 = control-ref of="Camera Settings"() -> (w7:refnum<vi>)
  n5 = call <vilib>:"Get Tab Control Refs.vi"("Page Index"=T10."Basic" ("Dashboard Tab"), "TabControl in"=w23) -> ("ControlsOnPage"=w12:refnum<vi>[])  [unwired: 9 in]
  n6 = call <vilib>:"Get Tab Control Refs.vi"("Page Index"=T10."Custom" ("Dashboard Tab"), "TabControl in"=w23) -> ("ControlsOnPage"=w22:refnum<vi>[])  [unwired: 9 in]
  n7 = Obtain Notifier(name (unnamed)="Window Mode", notification data type=TRUE) -> (notifier out=w20:refnum<notifier>)  [unwired: 2 in, 2 out]
  n8 = Obtain Notifier(name (unnamed)="Robot IP Update", notification data type="IP Addr" ("name (unnamed)")) -> (notifier out=w8:refnum<notifier>)  [unwired: 2 in, 2 out]
  n9 = Create User Event(user event datatype=w17) -> (user event=w14:refnum<user-event>)  [unwired: 1 in, 1 out]
  n10 = call "IMAQ Create"("Image Name"="Full Video Stream", "Image Type"=w4) -> ("New Image"=w2:T3)  [unwired: 2 in, 2 out]
  n11 = Build Array (concatenate)(w12, w22) -> (w21:refnum<vi>[])
  n12 = call "Handle Camera Configuration.vi"("CameraNameRef"=w6, "Display Name"=w1, "ClusterRef"=w7) -> ()  [unwired: 9 in]
  n13 = control-ref of="CheckList"() -> (w3:refnum<vi>)
  n14 = register-events(refnum<vi> refnum, w14) -> (reference out=w29:refnum<event-registration>, error out=w28:errorcluster)  [unwired: 2 in]
  n15 = while {
    tunnel: w21 -> [w42]
    tunnel: w8 -> [w40]
    tunnel: [w38] -> _
    tunnel: u32 1000 ("milliseconds to wait") -> [w37]
    tunnel: w14 -> [w34]
    i -> [w38]
    stop <- FALSE stop-if-true
    n16 = Wait on Notification(notifier=w40, timeout in ms (-1)=w37) -> (notification=w39:string, timed out?=w35:bool)  [unwired: 2 in, 2 out]
    n17 = Compound Arithmetic op=OR(invert w35) -> (w36:bool)
    n18 = case shown="True" w36 {
      tunnel: w42 -> [_ w45]
      tunnel: w39 -> [_ w44]
      tunnel: w34 -> [_ w43]
      frame False {
      }
      frame True {
        n19 = call <vilib>:"Bind Controls to SmartDashboard.vi"("RPC ref"=w43, "Bound Control Refs"=w45, "Server IP Address"=w44) -> ()  [unwired: 9 in]
      }
    }
  }
  n20 = while {
    tunnel: w1 -> [_]
    stop <- FALSE stop-if-true
    # "Maintain LimeLight connection"
    n21 = local read "Enable_Streaming_GUI"() -> (w46:bool)
    n22 = Wait (ms)(milliseconds to wait=u32 1000) -> ()  [unwired: 1 out]
    n23 = case shown="True" w46 {
      frame False {
      }
      frame True {
        w59 = "320x240 MJPEG 22 fps" ("String")
        w53 = "mjpg:http://10.42.65.11:5800"
        w58 = "/CameraPublisher/limelight/"
        # "manually configure the NT for a single LimeLight\ncamera in order to bypass WPILib's camera\nauto-detection which fails when the NTs are refreshed\nafter the code restarts on the roboRIO"
        n24 = Concatenate Strings("ip:http://", "10.42.65.11:5800" ("string")) -> (w61:string)
        n25 = Build Array(w53, w53) -> (w63:string[])
        n26 = Concatenate Strings(w58, "source") -> (w60:string)
        n27 = Concatenate Strings(w58, "description") -> (w64:string)
        n28 = Concatenate Strings(w58, "mode") -> (w65:string)
        n29 = Build Array(w59) -> (w67:string[])
        n30 = Concatenate Strings(w58, "streams") -> (w62:string)
        n31 = Concatenate Strings(w58, "modes") -> (w66:string)
        n32 = call-poly <vilib>:"NT Write Value.vi"("String"=w61, "Name"=w60) -> ()  [unwired: 9 in, 1 out]
        n33 = call-poly <vilib>:"NT Write Value.vi"("String"="limelight", "Name"=w64) -> ()  [unwired: 9 in, 1 out]
        n34 = call-poly <vilib>:"NT Write Value.vi"("String"=w59, "Name"=w65) -> ()  [unwired: 9 in, 1 out]
        n35 = call-poly <vilib>:"NT Write Value.vi"("String Array"=w63, "Name"=w62) -> ()  [unwired: 9 in, 1 out]
        n36 = call-poly <vilib>:"NT Write Value.vi"("String Array"=w67, "Name"=w66) -> ()  [unwired: 9 in, 1 out]
      }
    }
  }
  n37 = while {
    shift-right: [w78] -> _
    shift-left: _ -> [w131]
    shift-right: [w79] -> _
    shift-left: _ -> [w121]
    tunnel: w8 -> [_]
    stop <- FALSE stop-if-true
    # "Dynamic Overlays"
    n38 = To Long Integer(number="Reticule") -> (32bit integer=w112:i32)
    n39 = Wait (ms)(milliseconds to wait=u32 100) -> ()  [unwired: 1 out]
    n40 = Multiply(x=w112, y=2) -> (x*y=w111:i32)
    n41 = control-ref of="HUB_Ret_Left"() -> (w92:refnum<vi>)
    n42 = control-ref of="HUB_Ret_Right"() -> (w91:refnum<vi>)
    n43 = control-ref of="CARGO_Ret_Left"() -> (w77:refnum<vi>)
    n44 = control-ref of="CARGO_Ret_Right"() -> (w76:refnum<vi>)
    n45 = Increment(x=w111) -> (x+1=w98:i32)
    n46 = First Call?() -> (First Call?: T/F=w101:bool)
    n47 = Index Array(array=w121, index #1=w111, index #2=w98) -> (element #1=w115:i32, element #2=w123:i32)
    n48 = Or(x="Up", y="Down") -> (x .or. y?=w127:bool)
    n49 = Or(x="Left", y="Right") -> (x .or. y?=w117:bool)
    n50 = case shown="True" w101 {
      tunnel: [w142 w155] -> w78
      tunnel: w131 -> [w142 _]
      tunnel: w92 -> [_ w154]
      tunnel: w91 -> [_ w153]
      tunnel: w77 -> [_ w144]
      tunnel: w76 -> [_ w143]
      frame False {
      }
      frame True {
        n51 = property class="Bool (strict)"(reference=w154) -> ("Left"=w152:i32, "Top"=w151:i32)  [unwired: 1 in, 2 out]
        n52 = property class="Bool (strict)"(reference=w153) -> ("Left"=w150:i32, "Top"=w149:i32)  [unwired: 1 in, 2 out]
        n53 = property class="Bool (strict)"(reference=w144) -> ("Left"=w148:i32, "Top"=w147:i32)  [unwired: 1 in, 2 out]
        n54 = property class="Bool (strict)"(reference=w143) -> ("Left"=w146:i32, "Top"=w145:i32)  [unwired: 1 in, 2 out]
        n55 = Build Array(w152, w151, w150, w149, w148, w147, w146, w145) -> (w155:i32[])
      }
    }
    n56 = Bundle("HUB_Ret_Left"=w92, "HUB_Ret_Right"=w91, "CARGO_Ret_Left"=w77, "CARGO_Ret_Right"=w76) -> (w83:T13)  [unwired: 1 in]
    n57 = Decrement(x=w123) -> (x-1=w130:i32)
    n58 = Increment(x=w123) -> (x+1=w129:i32)
    n59 = Decrement(x=w115) -> (x-1=w120:i32)
    n60 = Increment(x=w115) -> (x+1=w119:i32)
    n61 = Select(t=w130, s="Up", f=w129) -> (s? t:f=w128:i32)
    n62 = Select(t=w120, s="Left", f=w119) -> (s? t:f=w118:i32)
    n63 = Select(t=w128, s=w127, f=w123) -> (s? t:f=w97:i32)
    n64 = Select(t=w118, s=w117, f=w115) -> (s? t:f=w116:i32)
    n65 = Replace Array Subset(array=w121, new element #1=w116, index #1=w111, new element #2=w97, index #2=w98) -> (w96:i32[])
    n66 = Current VI's Path() -> (path=w107:path)
    n67 = Strip Path(path=w107) -> (stripped path=w106:path)  [unwired: 1 out]
    n68 = Cluster To Array(cluster=w83) -> (array=w95:refnum<vi>[])
    n69 = Strip Path(path=w106) -> (stripped path=w105:path)  [unwired: 1 out]
    n70 = Array Size(array=w95) -> (size(s)=w94:i32)
    n71 = Build Path(base path=w105, name or relative path=path "reticule positions" ("XML File Path")) -> (appended path=w104:path)
    n72 = Multiply(x=2 ("dimension size"), y=w94) -> (x*y=w100:i32)
    n73 = Initialize Array(0, w100) -> (w90:i32[])
    n74 = call-poly <vilib>:"Read From XML File.vi"("XML File Path"=w104) -> ("error out"=w82:errorcluster, "XML Elements"=w103:string[])  [unwired: 8 in, 1 out]
    n75 = case shown="Error .." w82 {
      tunnel: w103 -> [w138 _]
      tunnel: w90 -> [w135 _]
      tunnel: [w134 i32[] [0, 0, 0, 0, 0, 0, 0, 0, 0, 0, 0, 0] ("value")] -> w80
      frame No Error {
        n76 = Index Array(array=w138, index=0) -> (element=w136:string)
        n77 = Unflatten From XML(xml string=w136, type=w135) -> (value=w134:i32[])  [unwired: 1 in, 1 out]
      }
      frame Error {
      }
    }
    n78 = First Call?() -> (First Call?: T/F=w122:bool)
    n79 = Select(t=w80, s=w122, f=w96) -> (s? t:f=w79:i32[])
    n80 = Add(x=w79, y=w78) -> (x+y=w81:i32[])
    n81 = Index Array(array=w81, index #1=0 ("index")) -> (element #1=w87:i32, element #2=w86:i32, element #3=w85:i32, element #4=w84:i32, element #5=w75:i32, element #6=w74:i32, element #7=w73:i32, element #8=w72:i32)  [unwired: 7 in]
    n82 = Unbundle(w83) -> ("HUB_Ret_Left"=w88:refnum<vi>, "HUB_Ret_Right"=w89:refnum<vi>, "CARGO_Ret_Left"=w71:refnum<vi>, "CARGO_Ret_Right"=w70:refnum<vi>)
    n83 = Flatten To XML(6:w79) -> (2:w109:string)
    n84 = call "EdgeTrigger.vi"("Input Signal"="Save") -> ("Rising Edge Trigger"=w68:bool)  [unwired: 2 out]
    n85 = case shown="True" w68 {
      tunnel: w109 -> [_ w141]
      tunnel: w104 -> [_ w140]
      frame False {
      }
      frame True {
        n86 = call-poly <vilib>:"Write to XML File.vi"("XML Input"=w141, "XML File Path"=w140) -> ()  [unwired: 7 in, 3 out]
      }
    }
    n87 = property class="Bool (strict)"(reference=w88, "Left"=w87, "Top"=w86) -> ()  [unwired: 1 in, 2 out]
    n88 = property class="Bool (strict)"(reference=w89, "Left"=w85, "Top"=w84) -> ()  [unwired: 1 in, 2 out]
    n89 = property class="Bool (strict)"(reference=w71, "Left"=w75, "Top"=w74) -> ()  [unwired: 1 in, 2 out]
    n90 = property class="Bool (strict)"(reference=w70, "Left"=w73, "Top"=w72) -> ()  [unwired: 1 in, 2 out]
  }
  n91 = while {
    tunnel: w9 -> [w185]
    tunnel: w1 -> [w169]
    tunnel: w2 -> [w167]
    stop <- FALSE stop-if-true
    w156 = u16 0 items=["Stop", "Record", "Playback Panel"] ("Rec Mode")
    # "Camera Feeds"
    n92 = First Call?() -> (First Call?: T/F=w163:bool)
    n93 = local read "NT Connection"() -> (w166:bool)
    n94 = call "Timer.vi"("Reset Timer"=w163) -> ("Time (ms)"=w162:u32)
    n95 = Greater?(x=w162, y=u32 5000) -> (0:w160:bool)
    n96 = Compound Arithmetic op=AND(w166, "Enable_Streaming_GUI", w160) -> (w165:bool)
    n97 = Bundle("Camera Name"="Camera Name", w169, "Saved DB Images Info"=w185) -> (w184:T14)  [unwired: 1 in]
    n98 = control-ref of="Camera Perf"() -> (w182:refnum<vi>)
    n99 = call <vilib>:"WPI_CameraRead MJPG for Dashboard_2.vi"("Camera Settings"="Camera Settings", "Rec Mode"=w156, "NT Connection"=w165, "Capture Info"=w184, "Image in"=w167) -> ("perf info"=w183:cluster{"Bandwidth (Mbps)":dbl, "fps":dbl}, "Active"=w168:bool, "Image\\ out"=w186:T3)  [unwired: 4 in]
    n100 = call <vilib>:"WPI_DashboardFormatPerf.vi"("Right Camera Perf"=cluster{"Bandwidth (Mbps)":dbl, "FPS":dbl} {"Bandwidth (Mbps)"=0.0, "FPS"=0.0}, "Performance"=w183, "String in"=w182) -> ()  [unwired: 9 in]
    n101 = case shown="True" w168 {
      tunnel: w186 -> [w197 w200]
      tunnel: [w197 w199] -> w181
      frame False {
        n102 = Wait Until Next ms Multiple(millisecond multiple=u32 500) -> ()  [unwired: 1 out]
      }
      frame True {
        # "image annotation etc."
        n103 = call "IMAQ Clear Overlay"("Image"=w200) -> ("Image Out"=w199:T3)  [unwired: 2 in, 8 out]
      }
    }
    n104 = call "IMAQ Rotate"("Angle (degrees)"=sgl 0.0, "Image Src"=w181) -> ("Image Dst Out"=w172:T3)  [unwired: 8 in, 1 out]
    n105 = call "IMAQ GetImageSize"("Image"=w172) -> ("Y Resolution"=w170:i32, "X Resolution"=w157:i32)  [unwired: 3 in, 1 out]
    n106 = To Double Precision Float(number=w157) -> (double precision float=w179:dbl)
    n107 = To Double Precision Float(number=w170) -> (double precision float=w178:dbl)
    n108 = Divide(x=w179, y=w178) -> (x/y=w177:dbl)
    n109 = Less?(x=w177, y=1.9) -> (x < y?=→"No_Secondary_Camera":bool)
    n110 = case shown="160, Default" w157 {
      tunnel: "Partial Video Stream" ("Image Name") -> [_ w196]
      tunnel: [w188 w195] -> w159
      tunnel: w172 -> [w188 w193]
      frame 320 {
        # "wide angle camera found"
      }
      frame 160, Default {
        w189 = T12 4 items=["Grayscale (U8)", "Grayscale (I16)", "Grayscale (SGL)", "Complex (CSG)", "RGB (U32)", "HSL (U32)", "RGB (U64)"] ("Image Type")
        # "no wide angle camera found"
        n111 = call "IMAQ Create"("Image Name"=w196, "Image Type"=w189) -> ("New Image"=w192:T3)  [unwired: 3 in, 1 out]
        n112 = call "IMAQ SetImageSize"("Y Resolution"=120, "X Resolution"=320, "Image"=w192) -> ("Image Out"=w194:T3)  [unwired: 2 in, 1 out]
        n113 = call "IMAQ ImageToImage 2"("Image Src (Small)"=w193, "Image Src (Large)"=w194) -> ("Image Dst Out"=w195:T3)  [unwired: 8 in, 1 out]
      }
    }
    "Combined Camera Feed" <- w159
  }
  n114 = while {
    tunnel: w8 -> [w205]
    tunnel: w20 -> [w202]
    stop <- FALSE stop-if-true
    # "Primary Indicators and Controls"
    n115 = Wait (ms)(milliseconds to wait=u32 50) -> ()  [unwired: 1 out]
    n116 = call <vilib>:"WPI_DashboardRetrieveStatusInfo.vi"("Binding Refnum"=w205, "Window Mode Notifier"=w202, "TCP Cnx"="TCP") -> ("Power and Errors"=w206:T17, "Robot Metrics"=w209:T18, "Status Info"=w210:T19, "Control Info"=w207:T20, "Robot Mode"=w204:T7, "Process?"=w208:bool)  [unwired: 3 in]
    "Mode" <- w204
    n117 = case shown="True" w208 {
      tunnel: w210 -> [_ w214]
      tunnel: w209 -> [_ w213]
      tunnel: w207 -> [_ w215]
      tunnel: w206 -> [_ w212]
      tunnel: w204 -> [_ _]
      frame False {
      }
      frame True {
        n118 = stacked-sequence {
          tunnel: w215 -> [_ _ _ _ _ _ _ _ _ _ _]
          tunnel: w214 -> [w220 _ _ _ _ _ _ _ _ _ _]
          tunnel: w213 -> [_ _ _ _ _ _ _ _ _ _ _]
          tunnel: w212 -> [_ _ _ _ _ _ _ _ _ _ _]
          frame #0 {
            # "general reporting"
            # "resource utilization"
            # "autonomous reporting"
            # "report robot status and resource utilization"
            n119 = Unbundle By Name(w220) -> ("Battery V"=→"Battery_Voltage_GUI":dbl)
            n120 = call-poly <vilib>:"NT Read Value.vi"("Name"="Battery_Critical") -> ("Boolean"=→"Battery_Critical_GUI":bool)  [unwired: 9 in, 1 out]
            n121 = call-poly <vilib>:"NT Read Value.vi"("Name"="Diverting_Power") -> ("Boolean"=→"Diverting_Power_GUI":bool)  [unwired: 9 in, 1 out]
            n122 = call-poly <vilib>:"NT Read Value.vi"("Name"="Electrical_Fault") -> ("Boolean"=→"Electrical_Fault_GUI":bool)  [unwired: 9 in, 1 out]
            n123 = call-poly <vilib>:"NT Read Value.vi"("Name"="CAN_Bus_Fault") -> ("Boolean"=→"CAN_Bus_Fault_GUI":bool)  [unwired: 9 in, 1 out]
            n124 = call-poly <vilib>:"NT Read Value.vi"("Name"="Control_Latency_Alarm") -> ("Boolean"=w249:bool)  [unwired: 9 in, 1 out]
            "Slow_Loop" <- w249
            n125 = call-poly <vilib>:"NT Read Value.vi"("Name"="Control_Loop_Time") -> ("Numeric"=w240:dbl)  [unwired: 9 in, 1 out]
            n126 = call-poly <vilib>:"NT Read Value.vi"("Name"="Pose_Loop_Time") -> ("Numeric"=w250:dbl)  [unwired: 9 in, 1 out]
            n127 = call-poly <vilib>:"NT Read Value.vi"("Name"="Compressor_On") -> ("Boolean"=→"Compressor_On_GUI":bool)  [unwired: 9 in, 1 out]
            n128 = call-poly <vilib>:"NT Read Value.vi"("Name"="Pressure_Vent") -> ("Boolean"=→"Pressure_Vent_GUI":bool)  [unwired: 9 in, 1 out]
            n129 = call-poly <vilib>:"NT Read Value.vi"("Name"="Pressure_Transducer") -> ("Numeric"=→"Pressure_Transducer_GUI":dbl)  [unwired: 9 in, 1 out]
            n130 = call-poly <vilib>:"NT Read Value.vi"("Name"="Pressure_Leak") -> ("Boolean"=→"Pressure_Leak_GUI":bool)  [unwired: 9 in, 1 out]
            n131 = To Unsigned Long Integer(number=w250) -> (unsigned 32bit integer=→"Pose_Loop_Time_GUI":u32)
            n132 = To Unsigned Long Integer(number=w240) -> (unsigned 32bit integer=→"Control_Loop_Time_GUI":u32)
            n133 = Select(t=u32 16711680 ("Numeric Text.Text Colors:Text Color"), s=w249, f=u32 4934475 ("Numeric Text.Text Colors:Text Color")) -> (s? t:f=w244:u32)
            n134 = property on="Control_Loop_Time_GUI" class="DigNum (strict)"("NumText.BG Color"=w244) -> ()  [unwired: 2 in, 2 out]
            n135 = call-poly <vilib>:"NT Read Value.vi"("Name"="Auto_Error") -> ("Boolean"=→"Auto_Error_GUI":bool)  [unwired: 9 in, 1 out]
            n136 = call-poly <vilib>:"NT Read Value.vi"("Name"="Robot_is_Autonomous") -> ("Boolean"=→"Robot_is_Autonomous_GUI_0" →"Robot_is_Autonomous_GUI_1" →"Robot_is_Autonomous_GUI_2":bool)  [unwired: 9 in, 1 out]
            n137 = local read "Dashboard Tab"() -> (w216:T1)
            n138 = case shown="\"Setup/Auto\"" w216 {
              frame "Checklist", Default {
              }
              frame "Setup/Auto" {
                n139 = call-poly <vilib>:"NT Read Value.vi"("Default Value"="No robot code versioning information...", "Name"="Robot_Code_Version") -> ("String"=→"Robot_Code_Version_GUI":string)  [unwired: 8 in, 1 out]
              }
            }
            n140 = local read "Dashboard Tab"() -> (w217:T1)
            n141 = To Double Precision Float(number=w217) -> (double precision float=w218:dbl)
            n142 = call "ReducedBWSendToNT.vim"("Value In"=w218, "NT Name"="Dashboard_Tab" ("Name")) -> ()  [unwired: 1 out]
          }
          frame #1 {
            # "targeting calibrations"
            # "targeting data"
            # "report robot pose and targeting data"
            n143 = call-poly <vilib>:"NT Read Value.vi"("Name"="Alliance_Color") -> ("Numeric"=w277:dbl)  [unwired: 9 in, 1 out]
            n144 = call-poly <vilib>:"NT Read Value.vi"("Default Value"=0.0, "Name"="Turret_H") -> ("Numeric"=w286:dbl)  [unwired: 8 in, 1 out]
            n145 = call-poly <vilib>:"NT Read Value.vi"("Default Value"=0.0, "Name"="Robot_H") -> ("Numeric"=w314:dbl)  [unwired: 8 in, 1 out]
            n146 = call-poly <vilib>:"NT Read Value.vi"("Default Value"=dbl[] [0.0, 0.0, 0.0, 0.0], "Name"="Targeting_Predictions") -> ("Numeric Array"=w280:dbl[])  [unwired: 8 in, 1 out]
            n147 = call-poly <vilib>:"NT Read Value.vi"("Default Value"=-1.0, "Name"="Robot_X") -> ("Numeric"=w312:dbl)  [unwired: 8 in, 1 out]
            "Robot_X" <- w312
            n148 = call-poly <vilib>:"NT Read Value.vi"("Default Value"=-1.0, "Name"="Robot_Y") -> ("Numeric"=w313:dbl)  [unwired: 8 in, 1 out]
            "Robot_Y" <- w313
            n149 = call-poly <vilib>:"NT Read Value.vi"("Default Value"=30.0, "Name"="Robot_Width_Bumpers") -> ("Numeric"=w271:dbl)  [unwired: 8 in, 1 out]
            n150 = call-poly <vilib>:"NT Read Value.vi"("Default Value"=30.0, "Name"="Robot_Length_Bumpers") -> ("Numeric"=w272:dbl)  [unwired: 8 in, 1 out]
            n151 = To Unsigned Word Integer(number=w277) -> (unsigned 16bit integer=w297:u16)
            n152 = feedback #1(w297) -> (w293:u16)
            n153 = feedback-in #1(w297) -> ()
            n154 = Not Equal?(x=w297, y=w293) -> (x != y?=w295:bool)
            n155 = feedback #2("Field Map") -> (w298:u16)
            n156 = feedback-in #2("Field Map") -> ()
            n157 = Not Equal?(x="Field Map", y=w298) -> (x != y?=w300:bool)
            n158 = Quotient & Remainder(x=w286, y=360.0) -> (x-y*floor(x/y)=→"Turret_H_GUI":dbl)  [unwired: 1 out]
            n159 = Quotient & Remainder(x=w314, y=360.0) -> (x-y*floor(x/y)=→"Robot_H_GUI":dbl)  [unwired: 1 out]
            n160 = First Call?() -> (First Call?: T/F=w294:bool)
            n161 = call "EdgeTrigger.vi"("Input Signal"="Export_Robot_Pose") -> ("Rising Edge Trigger"=w301:bool)  [unwired: 2 out]
            n162 = Compound Arithmetic op=OR(w295, w294, w300) -> (w296:bool)
            n163 = case shown="True" w296 {
              tunnel: w297 -> [_ w327]
              tunnel: "Field Map" -> [_ w325]
              frame False {
              }
              frame True {
                # "load and display a field map"
                n164 = To Long Integer(number=w325) -> (32bit integer=w323:i32)
                n165 = Current VI's Path() -> (path=w330:path)
                n166 = Strip Path(path=w330) -> (stripped path=w329:path)  [unwired: 1 out]
                n167 = Strip Path(path=w329) -> (stripped path=w326:path)  [unwired: 1 out]
                n168 = List Folder(path=w326, pattern="*map*.png") -> (filenames=w324:string[])  [unwired: 2 in, 3 out]
                n169 = Index Array(array=w324, index=w323) -> (element=w322:string)
                n170 = property on="Field Map" class="Ring (strict)"("Strings []"=w324) -> ()  [unwired: 2 in, 2 out]
                n171 = Build Path(base path=w326, name or relative path=w322) -> (appended path=w328:path)
                n172 = call <vilib>:"Read PNG File.vi"("path to PNG file"=w328) -> ("error out"=w332:errorcluster, "image data"=w331:T21)  [unwired: 8 in, 1 out]
                n173 = case shown="No Error" w332 {
                  tunnel: w331 -> [w335 _]
                  tunnel: w327 -> [w350 _]
                  frame No Error {
                    w345 = T12 4 items=["Grayscale (U8)", "Grayscale (I16)", "Grayscale (SGL)", "Complex (CSG)", "RGB (U32)", "HSL (U32)", "RGB (U64)", "Grayscale (U16)"] ("Image Type")
                    w365 = T12 4 items=["Grayscale (U8)", "Grayscale (I16)", "Grayscale (SGL)", "Complex (CSG)", "RGB (U32)", "HSL (U32)", "RGB (U64)", "Grayscale (U16)"] ("Image Type")
                    n174 = call <vilib>:"Unflatten Pixmap.vi"("image data"=w335) -> ("24-bit pixmap"=w364:u32[][])  [unwired: 4 in, 6 out]
                    n175 = call <vilib>:"Unflatten Pixmap.vi"("image data"=w335) -> ("24-bit pixmap"=w344:u32[][])  [unwired: 4 in, 6 out]
                    n176 = property on="Robot Pose 1" class="XYGraph (strict)"() -> ("Width"=w368:u32, "Height"=w367:u32)  [unwired: 2 in, 2 out]
                    n177 = property on="Robot Pose 2" class="XYGraph (strict)"() -> ("Width"=w348:u32, "Height"=w347:u32)  [unwired: 2 in, 2 out]
                    n178 = call "IMAQ Create"("Image Name"="field1", "Image Type"=w365) -> ("New Image"=w363:T3)  [unwired: 3 in, 1 out]
                    n179 = call "IMAQ Create"("Image Name"="field2", "Image Type"=w345) -> ("New Image"=w343:T3)  [unwired: 3 in, 1 out]
                    n180 = Equal?(x=w350, y=WPI_DriverStationAllianceInfo."Red" ("x")) -> (x = y?=w352:bool)
                    n181 = call "IMAQ ArrayToColorImage"("Image Pixels (U32)"=w364, "Image"=w363) -> ("Image Out"=w362:T3)  [unwired: 3 in, 1 out]
                    n182 = call "IMAQ ArrayToColorImage"("Image Pixels (U32)"=w344, "Image"=w343) -> ("Image Out"=w342:T3)  [unwired: 3 in, 1 out]
                    n183 = To Long Integer(number=w368) -> (32bit integer=w358:i32)
                    n184 = To Long Integer(number=w367) -> (32bit integer=w359:i32)
                    n185 = To Long Integer(number=w348) -> (32bit integer=w338:i32)
                    n186 = To Long Integer(number=w347) -> (32bit integer=w339:i32)
                    n187 = call "IMAQ Resample"("X Resolution"=w358, "Y Resolution"=w359, "Image Src"=w362) -> ("Image Dst Out"=w357:T3)  [unwired: 7 in, 1 out]
                    n188 = call "IMAQ Resample"("X Resolution"=w338, "Y Resolution"=w339, "Image Src"=w342) -> ("Image Dst Out"=w337:T3)  [unwired: 7 in, 1 out]
                    n189 = Select(t=180.0, s=w352, f=0.0) -> (s? t:f=w355:dbl)
                    n190 = To Single Precision Float(number=w355) -> (single precision float=w333:sgl)
                    n191 = call "IMAQ Rotate"("Angle (degrees)"=w333, "Image Src"=w357) -> ("Image Dst Out"=w356:T3)  [unwired: 8 in, 1 out]
                    n192 = call "IMAQ Rotate"("Angle (degrees)"=w333, "Image Src"=w337) -> ("Image Dst Out"=w336:T3)  [unwired: 8 in, 1 out]
                    n193 = call "IMAQ ColorImageToArray"("Image"=w356) -> ("Image Pixels (U32)"=w361:u32[][])  [unwired: 3 in, 2 out]
                    n194 = call "IMAQ ColorImageToArray"("Image"=w336) -> ("Image Pixels (U32)"=w341:u32[][])  [unwired: 3 in, 2 out]
                    n195 = call <vilib>:"Flatten Pixmap.vi"("24-bit pixmap"=w361) -> ("image data"=w360:T21)  [unwired: 10 in]
                    n196 = call <vilib>:"Flatten Pixmap.vi"("24-bit pixmap"=w341) -> ("image data"=w340:T21)  [unwired: 10 in]
                    n197 = call <vilib>:"Draw Flattened Pixmap.vi"("image data"=w360) -> ("new picture"=w349:picture)  [unwired: 8 in]
                    n198 = call <vilib>:"Draw Flattened Pixmap.vi"("image data"=w340) -> ("new picture"=w334:picture)  [unwired: 8 in]
                    n199 = property on="Robot Pose 1" class="XYGraph (strict)"("PlotImages.Back"=w349) -> ()  [unwired: 2 in, 2 out]
                    n200 = property on="Robot Pose 2" class="XYGraph (strict)"("PlotImages.Back"=w334) -> ()  [unwired: 2 in, 2 out]
                  }
                  frame Error {
                  }
                }
              }
            }
            n201 = case shown="True" w301 {
              frame False {
              }
              frame True {
                # "export the current robot pose data"
                n202 = Get Date/Time In Seconds() -> (seconds since 1Jan1904=w382:timestamp)
                n203 = Format Date/Time String(time format string (%c)="%Y-%m-%d_%H-%M", seconds (now)=w382) -> (date/time string=w380:string)  [unwired: 1 in]
                n204 = Concatenate Strings("robot pose data " ("string"), w380) -> (w378:string)
                n205 = Current VI's Path() -> (path=w377:path)
                n206 = String To Path(string=w378) -> (path=w374:path)
                n207 = Strip Path(path=w377) -> (stripped path=w376:path)  [unwired: 1 out]
                n208 = Strip Path(path=w376) -> (stripped path=w375:path)  [unwired: 1 out]
                n209 = Build Path(base path=w375, name or relative path=w374) -> (appended path=w373:path)
                n210 = invoke on="Robot Pose 1" class="XYGraph (strict)" method="Export Image"("FileType"=enum32{"BMP", "EPS", "EMF", "PICT"}."BMP" ("File Type"), "Target"=enum32{"File", "Clipboard"}."File", "Path"=w373, "HideGrid"=TRUE ("Hide Grid"), "Overwrite"=TRUE ("Always Overwrite")) -> ()  [unwired: 3 in, 8 out]
              }
            }
            n211 = call "RenderRobotPose.vi"("Robot X (in)"=w312, "Robot Width (in)"=w271, "Robot Length (in)"=w272, "Buffer Time (min)"=0.5, "Robot Y (in)"=w313, "Targeting Predictions"=w280, "Robot Heading (deg)"=w314, "Turret Heading (deg)"=w286, "Robot Enabled"=TRUE, "Reset"="Clear_Robot_Pose_Display") -> ("Robot Pose"=→"Robot Pose 2" →"Robot Pose 1":cluster{dbl[], dbl[]}[])  [unwired: 5 in]
            n212 = call-poly <vilib>:"NT Read Value.vi"("Name"="LL_Valid") -> ("Boolean"=→"LL_Valid":bool)  [unwired: 9 in, 1 out]
            n213 = call-poly <vilib>:"NT Read Value.vi"("Name"="Vision_Fault") -> ("Boolean"=→"Vision_Fault_GUI":bool)  [unwired: 9 in, 1 out]
            n214 = call-poly <vilib>:"NT Read Value.vi"("Name"="Range_To_Target") -> ("Numeric"=→"Range_To_Target_GUI" →"Range_To_Target_GUI_Small":dbl)  [unwired: 9 in, 1 out]
            n215 = call-poly <vilib>:"NT Read Value.vi"("Name"="Angle_To_Target") -> ("Numeric"=→"Angle_To_Target_GUI" →"Angle_To_Target_GUI_Small":dbl)  [unwired: 9 in, 1 out]
            n216 = local read "No_Secondary_Camera"() -> (w264:bool)
            n217 = local read "Intake_Intaking_GUI"() -> (w262:bool)
            n218 = local read "Dashboard Tab"() -> (w256:T1)
            n219 = Not(x=w264) -> (.not. x?=w263:bool)
            n220 = And(x=w263, y=w262) -> (x .and. y?=w261:bool)
            n221 = Not(x=w261) -> (.not. x?=w260:bool)
            n222 = case shown="\"Setup/Auto\"" w256 {
              frame "Checklist", Default {
              }
              frame "Setup/Auto" {
                n223 = call-poly <vilib>:"NT Read Value.vi"("Name"="Current_HUB_Height_Offset") -> ("Numeric"=w315:dbl)  [unwired: 9 in, 1 out]
                "Current_HUB_Height_Offset_GUI" <- w315
                n224 = feedback #3(0.0 ("Numeric")) -> (w317:dbl)
                n225 = feedback-in #3(w315) -> ()
                n226 = Not Equal?(x=w315, y=w317) -> (x != y?=w318:bool)
                n227 = case shown="True" w318 {
                  tunnel: w315 -> [_ w320]
                  frame False {
                  }
                  frame True {
                    n228 = property on="New_HUB_Height_Offset_GUI" class="DigNum (strict)"("Value"=w320) -> ()  [unwired: 2 in, 2 out]
                  }
                }
              }
            }
            n229 = property on="Robot Pose 2" class="XYGraph (strict)"("Visible"=w260) -> ()  [unwired: 2 in, 2 out]
            n230 = call "ReducedBWSendToNT.vim"("Value In"="New_HUB_Height_Offset_GUI", "NT Name"="New_HUB_Height_Offset" ("Name")) -> ()  [unwired: 1 out]
            n231 = call "ReducedBWSendToNT.vim"("Value In"="Apply_New_HUB_Height_Offset_GUI", "NT Name"="Apply_New_HUB_Height_Offset" ("Name")) -> ()  [unwired: 1 out]
          }
          frame #2 {
            # "driver control configuration"
            # "robot configuration"
            # "robot and driver control configuration"
            n232 = local read "Dashboard Tab"() -> (w383:T1)
            n233 = case shown="\"Setup/Auto\"" w383 {
              frame "Checklist", Default {
              }
              frame "Setup/Auto" {
                n234 = call-poly <vilib>:"NT Read Value.vi"("Default Value"="No robot profile...", "Name"="Robot_Profile") -> ("String"=→"Robot_Profile_GUI":string)  [unwired: 8 in, 1 out]
              }
            }
            n235 = Build Array("N/A") -> (w394:string[])
            n236 = And(x="Calibrate_Joysticks_GUI", y="Arm_Calibrate_Joysticks") -> (x .and. y?=w384:bool)
            n237 = To Double Precision Float(number="Driver Profile (1)") -> (double precision float=w387:dbl)
            n238 = call-poly <vilib>:"NT Read Value.vi"("Default Value"=w394, "Name"="Legal_Drivers") -> ("String Array"=w393:string[])  [unwired: 8 in, 1 out]
            "Legal_Drivers_GUI" <- w393
            n239 = Not(x="Arm_Calibrate_Joysticks") -> (.not. x?=w396:bool)
            n240 = call "ReducedBWSendToNT.vim"("Value In"=w387, "NT Name"="Selected_Driver" ("Name")) -> ()  [unwired: 1 out]
            n241 = property on="Driver Profile (1)" class="Ring (strict)"("Strings []"=w393) -> ()  [unwired: 2 in, 2 out]
            n242 = call "ReducedBWSendToNT.vim"("Value In"=w384, "NT Name"="Calibrate_Joysticks" ("Name")) -> ()  [unwired: 1 out]
            n243 = Select(t=cluster{u32, u32}[] [{11776947, 16448250}, {16448250, 16448250}] ("Colors [4]"), s=w396, f=cluster{u32, u32}[] [{6618880, 16448250}, {16448250, 16448250}] ("Colors [4]")) -> (s? t:f=w397:cluster{u32, u32}[])
            n244 = property on="Calibrate_Joysticks_GUI" class="Bool"("Colors [4]"=w397) -> ()  [unwired: 2 in, 2 out]
          }
          frame #3 {
            # "configure auto play"
            # "set robot pose"
            # "autonomous configuration"
            n245 = call "ReducedBWSendToNT.vim"("Value In"="Manual_Start_X", "NT Name"="Manual_Start_X" ("Name")) -> ()  [unwired: 1 out]
            n246 = call "ReducedBWSendToNT.vim"("Value In"="Manual_Start_Y", "NT Name"="Manual_Start_Y" ("Name")) -> ()  [unwired: 1 out]
            n247 = call "ReducedBWSendToNT.vim"("Value In"="Manual_Start_H", "NT Name"="Manual_Start_H" ("Name")) -> ()  [unwired: 1 out]
            n248 = call "ReducedBWSendToNT.vim"("Value In"="Disable_Fusion_While_Autonomous", "NT Name"="Disable_Fusion_While_Autonomous" ("Name")) -> ()  [unwired: 1 out]
            n249 = call "ReducedBWSendToNT.vim"("Value In"="Disable_Fusion_While_Disabled", "NT Name"="Disable_Fusion_While_Disabled" ("Name")) -> ()  [unwired: 1 out]
            n250 = call "ReducedBWSendToNT.vim"("Value In"="Push_Robot_Start_GUI", "NT Name"="Push_Robot_Start" ("Name")) -> ()  [unwired: 1 out]
            n251 = local read "Dashboard Tab"() -> (w402:T1)
            n252 = case shown="\"Setup/Auto\"" w402 {
              frame "Checklist", Default {
              }
              frame "Setup/Auto" {
                w426 = "Waiting for connection..." ("Default Value")
                n253 = Build Array("N/A") -> (w429:string[])
                n254 = call-poly <vilib>:"NT Read Value.vi"("Default Value"=w426, "Name"="Auto_Playbook") -> ("String"=→"Auto_Playbook_GUI":string)  [unwired: 8 in, 1 out]
                n255 = call-poly <vilib>:"NT Read Value.vi"("Default Value"=w426, "Name"="Auto_Path_Suffix") -> ("String"=→"Auto_Suffix_GUI":string)  [unwired: 8 in, 1 out]
                n256 = call-poly <vilib>:"NT Read Value.vi"("Default Value"=w429, "Name"="Legal_Auto_Plays") -> ("String Array"=w430:string[])  [unwired: 8 in, 1 out]
                n257 = property on="Select Autonomous Play" class="Ring (strict)"("Strings []"=w430) -> ()  [unwired: 2 in, 2 out]
              }
            }
            n258 = To Double Precision Float(number="Select Autonomous Play") -> (double precision float=w406:dbl)
            n259 = call "ReducedBWSendToNT.vim"("Value In"="Auto_Test_Mode_GUI", "NT Name"="Auto_Test_Mode" ("Name")) -> ()  [unwired: 1 out]
            n260 = call "ReducedBWSendToNT.vim"("Value In"="Auto_Delay_GUI", "NT Name"="Auto_Delay" ("Name")) -> ()  [unwired: 1 out]
            n261 = call "ReducedBWSendToNT.vim"("Value In"="Force_Human_Control_GUI", "NT Name"="Force_Human_Control" ("Name")) -> ()  [unwired: 1 out]
            n262 = call "ReducedBWSendToNT.vim"("Value In"=w406, "NT Name"="Selected_Auto_Play" ("Name")) -> ()  [unwired: 1 out]
            n263 = call "ReducedBWSendToNT.vim"("Value In"="Refresh_Auto_Play_List_GUI", "NT Name"="Refresh_Auto_Play_List" ("Name")) -> ()  [unwired: 1 out]
          }
          frame #4 {
            w447 = cluster{u32, u32}[] [{15663313, 16448250}, {16448250, 16448250}] ("Un-selected Color")
            w450 = cluster{u32, u32}[] [{9567230, 16448250}, {16448250, 16448250}] ("Un-selected Color")
            # "shooter state controller"
            # "master state controller"
            # "state indicators"
            n264 = call-poly <vilib>:"NT Read Value.vi"("Name"="Confirmed_States") -> ("Boolean Array"=w473:bool[])  [unwired: 9 in, 1 out]
            n265 = call-poly <vilib>:"NT Read Value.vi"("Default Value"=bool[] [FALSE, TRUE], "Name"="Disallowed_States") -> ("Boolean Array"=w474:bool[])  [unwired: 8 in, 1 out]
            n266 = Index Array(array=w474, index #1=0 ("index")) -> (element #1=w476:bool, element #2=w437:bool)  [unwired: 1 in]
            n267 = Index Array(array=w473, index #1=0 ("index")) -> (element #1=w475:bool, element #2=w449:bool)  [unwired: 1 in]
            n268 = Not(x=w437) -> (.not. x?=→"Arm_Climber":bool)
            n269 = call "ButtonColorChooser.vi"("Un-selected Color"=w450, "Disallowed"=w476, "Confirmed"=w475) -> ("Final Color"=w477:cluster{u32, u32}[])  [unwired: 8 in]
            n270 = call "ButtonColorChooser.vi"("Un-selected Color"=w450, "Disallowed"=w437, "Confirmed"=w449) -> ("Final Color"=w478:cluster{u32, u32}[])  [unwired: 8 in]
            n271 = property on="Master_State_0_Indicator" class="Bool (strict)"("Colors [4]"=w477) -> ()  [unwired: 2 in, 2 out]
            n272 = property on="Master_State_1_Indicator" class="Bool (strict)"("Colors [4]"=w478) -> ()  [unwired: 2 in, 2 out]
            n273 = call-poly <vilib>:"NT Read Value.vi"("Name"="Confirmed_Shooter_States") -> ("Boolean Array"=w455:bool[])  [unwired: 9 in, 1 out]
            n274 = call-poly <vilib>:"NT Read Value.vi"("Name"="Disallowed_Shooter_States") -> ("Boolean Array"=w456:bool[])  [unwired: 9 in, 1 out]
            n275 = Index Array(array=w456, index #1=0 ("index")) -> (element #1=w458:bool, element #2=w461:bool, element #3=w465:bool, element #4=w468:bool, element #5=w445:bool)  [unwired: 4 in]
            n276 = Index Array(array=w455, index #1=0 ("index")) -> (element #1=w457:bool, element #2=w460:bool, element #3=w462:bool, element #4=w467:bool, element #5=w446:bool)  [unwired: 4 in]
            n277 = call "ButtonColorChooser.vi"("Un-selected Color"=w447, "Disallowed"=w458, "Confirmed"=w457) -> ("Final Color"=w459:cluster{u32, u32}[])  [unwired: 8 in]
            n278 = call "ButtonColorChooser.vi"("Un-selected Color"=w447, "Disallowed"=w461, "Confirmed"=w460) -> ("Final Color"=w464:cluster{u32, u32}[])  [unwired: 8 in]
            n279 = call "ButtonColorChooser.vi"("Un-selected Color"=w447, "Disallowed"=w465, "Confirmed"=w462) -> ("Final Color"=w463:cluster{u32, u32}[])  [unwired: 8 in]
            n280 = call "ButtonColorChooser.vi"("Un-selected Color"=w447, "Disallowed"=w468, "Confirmed"=w467) -> ("Final Color"=w466:cluster{u32, u32}[])  [unwired: 8 in]
            n281 = call "ButtonColorChooser.vi"("Un-selected Color"=w447, "Disallowed"=w445, "Confirmed"=w446) -> ("Final Color"=w448:cluster{u32, u32}[])  [unwired: 8 in]
            n282 = property on="Shooter_State_0_Indicator" class="Bool (strict)"("Colors [4]"=w459) -> ()  [unwired: 2 in, 2 out]
            n283 = property on="Shooter_State_2_Indicator" class="Bool (strict)"("Colors [4]"=w463) -> ()  [unwired: 2 in, 2 out]
            n284 = property on="Shooter_State_3_Indicator" class="Bool (strict)"("Colors [4]"=w466) -> ()  [unwired: 2 in, 2 out]
            n285 = property on="Shooter_State_1_Indicator" class="Bool (strict)"("Colors [4]"=w464) -> ()  [unwired: 2 in, 2 out]
            n286 = property on="Shooter_State_4_Indicator" class="Bool (strict)"("Colors [4]"=w448) -> ()  [unwired: 2 in, 2 out]
            "Shooter_State_0_Indicator" <- FALSE ("Targeting_Computer_Indicator")
            "Shooter_State_1_Indicator" <- FALSE ("Mode_Shooter_1_Indicator")
            "Shooter_State_2_Indicator" <- FALSE ("Mode_Shooter_2_Indicator")
            "Shooter_State_3_Indicator" <- FALSE ("Mode_Shooter_3_Indicator")
            "Shooter_State_4_Indicator" <- FALSE ("Mode_Shooter_4_Indicator")
            "Master_State_0_Indicator" <- FALSE ("Master_State_0_Indicator")
            "Master_State_1_Indicator" <- FALSE ("Master_State_1_Indicator")
          }
          frame #5 {
            # "actuator test interlocks"
            # "emergency overrides"
            # "emergency overrides and interlocks"
            n287 = call-poly <vilib>:"NT Read Value.vi"("Name"="Robot_in_Safety_Override") -> ("Boolean"=w479:bool)  [unwired: 9 in, 1 out]
            n288 = call "EdgeTrigger.vi"("Input Signal"=w479) -> ("All Edge Trigger"=w480:bool)  [unwired: 2 out]
            n289 = case shown="True" w480 {
              tunnel: w479 -> [_ w508]
              frame False {
              }
              frame True {
                n290 = property on="Master_Safety_Override_1" class="Bool (strict)"("Value"=w508) -> ()  [unwired: 2 in, 2 out]
              }
            }
            n291 = call "ReducedBWSendToNT.vim"("Value In"="Clear_Errors_GUI", "NT Name"="Clear_Errors" ("Name")) -> ()  [unwired: 1 out]
            n292 = call "ReducedBWSendToNT.vim"("Value In"="Auto_Indexing_Override_GUI", "NT Name"="Auto_Indexing_Override" ("Name")) -> ()  [unwired: 1 out]
            n293 = call "ReducedBWSendToNT.vim"("Value In"="Super_Test_Mode_GUI", "NT Name"="Super_Test_Mode" ("Name")) -> ()  [unwired: 1 out]
            n294 = call "ReducedBWSendToNT.vim"("Value In"="Camera_Override_GUI", "NT Name"="Camera_Override" ("Name")) -> ()  [unwired: 1 out]
            n295 = call "ReducedBWSendToNT.vim"("Value In"="Field_Oriented_Override_GUI", "NT Name"="Field_Oriented_Override" ("Name")) -> ()  [unwired: 1 out]
            n296 = call "ReducedBWSendToNT.vim"("Value In"="Auto_Target_Override_GUI", "NT Name"="Auto_Target_Override" ("Name")) -> ()  [unwired: 1 out]
            n297 = call "ReducedBWSendToNT.vim"("Value In"="Master_Safety_Override_1", "NT Name"="Master_Safety_Override" ("Name")) -> ()  [unwired: 1 out]
            n298 = property on="Actuator Testing" class="Ring (strict)"() -> ("RingText.Text"=w491:string)  [unwired: 2 in, 2 out]
            n299 = Build Array("No_Test") -> (w507:string[])
            n300 = call "ReducedBWSendToNT.vim"("Value In"="Free_Tuning_Variable_GUI", "NT Name"="Free_Tuning_Variable" ("Name")) -> ()  [unwired: 1 out]
            n301 = call-poly <vilib>:"NT Read Value.vi"("Default Value"=w507, "Name"="Legal_Actuator_Names") -> ("String Array"=w506:string[])  [unwired: 8 in, 1 out]
            n302 = call "ReducedBWSendToNT.vim"("Value In"=w491, "NT Name"="Test_Actuator_Name" ("Name")) -> ()  [unwired: 1 out]
            n303 = call "ReducedBWSendToNT.vim"("Value In"="Test_Actuator_Value_GUI", "NT Name"="Test_Actuator_Value" ("Name")) -> ()  [unwired: 1 out]
            n304 = call "ReducedBWSendToNT.vim"("Value In"="Test_Actuator_Period_GUI", "NT Name"="Test_Actuator_Period" ("Name")) -> ()  [unwired: 1 out]
            n305 = property on="Actuator Testing" class="Ring (strict)"("Strings []"=w506) -> ()  [unwired: 2 in, 2 out]
          }
          frame #6 {
            # "drivebase subsytem"
            n306 = call "SwerveModuleReadData.vi"("NT Name (Errors)"="Swerve_1_Errors", "NT Name (Details)"="Swerve_1_Details" ("NT Name (Tune)")) -> ("Shifter State"=→"Swerve_1_Shifter_State":string, "Drive Velocity"=→"Swerve_1_Drive_Velocity":dbl, "Drive Temperature"=→"Swerve_1_Drive_Temperature":dbl, "Azimuth Position"=→"Swerve_1_Azimuth_Position":dbl, "Shifter Failure"=w558:T22, "Drive Overheating"=w560:T22, "Azimuth Fault"=w559:T22)  [unwired: 3 in]
            n307 = call "SwerveModuleReadData.vi"("NT Name (Errors)"="Swerve_0_Errors", "NT Name (Details)"="Swerve_0_Details" ("NT Name (Tune)")) -> ("Shifter State"=→"Swerve_0_Shifter_State":string, "Drive Velocity"=→"Swerve_0_Drive_Velocity":dbl, "Drive Temperature"=→"Swerve_0_Drive_Temperature":dbl, "Azimuth Position"=→"Swerve_0_Azimuth_Position":dbl, "Shifter Failure"=w566:T22, "Drive Overheating"=w574:T22, "Azimuth Fault"=w570:T22)  [unwired: 3 in]
            n308 = call-poly <vilib>:"NT Read Value.vi"("Name"="Field_Oriented") -> ("Boolean"=→"Field_Oriented_GUI":bool)  [unwired: 9 in, 1 out]
            n309 = call-poly <vilib>:"NT Read Value.vi"("Name"="IMU_Failure") -> ("Boolean"=→"IMU_Failure_GUI":bool)  [unwired: 9 in, 1 out]
            n310 = call "SwerveModuleReadData.vi"("NT Name (Errors)"="Swerve_2_Errors", "NT Name (Details)"="Swerve_2_Details" ("NT Name (Tune)")) -> ("Shifter State"=→"Swerve_2_Shifter_State":string, "Drive Velocity"=→"Swerve_2_Drive_Velocity":dbl, "Drive Temperature"=→"Swerve_2_Drive_Temperature":dbl, "Azimuth Position"=→"Swerve_2_Azimuth_Position":dbl, "Shifter Failure"=w553:T22, "Drive Overheating"=w555:T22, "Azimuth Fault"=w554:T22)  [unwired: 3 in]
            n311 = call "SwerveModuleReadData.vi"("NT Name (Errors)"="Swerve_3_Errors", "NT Name (Details)"="Swerve_3_Details" ("NT Name (Tune)")) -> ("Shifter State"=→"Swerve_3_Shifter_State":string, "Drive Velocity"=→"Swerve_3_Drive_Velocity":dbl, "Drive Temperature"=→"Swerve_3_Drive_Temperature":dbl, "Azimuth Position"=→"Swerve_3_Azimuth_Position":dbl, "Shifter Failure"=w548:T22, "Drive Overheating"=w550:T22, "Azimuth Fault"=w549:T22)  [unwired: 3 in]
            n312 = Unbundle(w560) -> ("Boolean"=w546:bool, "Numeric Text.Text Colors:Text Color"=w543:u32)
            n313 = Unbundle(w559) -> ("Boolean"=w547:bool, "Numeric Text.Text Colors:Text Color"=w544:u32)
            n314 = Unbundle(w574) -> ("Boolean"=w572:bool, "Numeric Text.Text Colors:Text Color"=w573:u32)
            n315 = Unbundle(w570) -> ("Boolean"=w569:bool, "Numeric Text.Text Colors:Text Color"=w567:u32)
            n316 = Unbundle(w558) -> ("Boolean"=w545:bool, "Numeric Text.Text Colors:Text Color"=w538:u32)
            n317 = Unbundle(w555) -> ("Boolean"=w536:bool, "Numeric Text.Text Colors:Text Color"=w534:u32)
            n318 = Unbundle(w566) -> ("Boolean"=w564:bool, "Numeric Text.Text Colors:Text Color"=w565:u32)
            n319 = Unbundle(w554) -> ("Boolean"=w537:bool, "Numeric Text.Text Colors:Text Color"=w535:u32)
            n320 = Unbundle(w550) -> ("Boolean"=w525:bool, "Numeric Text.Text Colors:Text Color"=w524:u32)
            n321 = Unbundle(w549) -> ("Boolean"=w526:bool, "Numeric Text.Text Colors:Text Color"=w527:u32)
            n322 = Unbundle(w553) -> ("Boolean"=w529:bool, "Numeric Text.Text Colors:Text Color"=w528:u32)
            n323 = Unbundle(w548) -> ("Boolean"=w518:bool, "Numeric Text.Text Colors:Text Color"=w519:u32)
            n324 = property on="Swerve_0_Azimuth_Position" class="DigNum (strict)"("NumText.BG Color"=w567) -> ()  [unwired: 2 in, 2 out]
            n325 = property on="Swerve_0_Drive_Temperature" class="DigNum (strict)"("NumText.BG Color"=w573) -> ()  [unwired: 2 in, 2 out]
            n326 = property on="Swerve_0_Shifter_State" class="Str"("Text.BG Color"=w565) -> ()  [unwired: 2 in, 2 out]
            n327 = property on="Swerve_1_Azimuth_Position" class="DigNum (strict)"("NumText.BG Color"=w544) -> ()  [unwired: 2 in, 2 out]
            n328 = property on="Swerve_1_Drive_Temperature" class="DigNum (strict)"("NumText.BG Color"=w543) -> ()  [unwired: 2 in, 2 out]
            n329 = property on="Swerve_1_Shifter_State" class="Str"("Text.BG Color"=w538) -> ()  [unwired: 2 in, 2 out]
            n330 = property on="Swerve_2_Azimuth_Position" class="DigNum (strict)"("NumText.BG Color"=w535) -> ()  [unwired: 2 in, 2 out]
            n331 = property on="Swerve_2_Drive_Temperature" class="DigNum (strict)"("NumText.BG Color"=w534) -> ()  [unwired: 2 in, 2 out]
            n332 = property on="Swerve_2_Shifter_State" class="Str"("Text.BG Color"=w528) -> ()  [unwired: 2 in, 2 out]
            n333 = property on="Swerve_3_Azimuth_Position" class="DigNum (strict)"("NumText.BG Color"=w527) -> ()  [unwired: 2 in, 2 out]
            n334 = property on="Swerve_3_Drive_Temperature" class="DigNum (strict)"("NumText.BG Color"=w524) -> ()  [unwired: 2 in, 2 out]
            n335 = property on="Swerve_3_Shifter_State" class="Str"("Text.BG Color"=w519) -> ()  [unwired: 2 in, 2 out]
            n336 = Build Array(w564, w545, w529, w518) -> (→"Swerve_Shifter_Failure_Array":bool[])
            n337 = Build Array(w569, w547, w537, w526) -> (→"Swerve_Azimuth_Fault_Array":bool[])
            n338 = Build Array(w572, w546, w536, w525) -> (→"Swerve_Overheating_Array":bool[])
            n339 = local read "Dashboard Tab"() -> (w509:T1)
            n340 = case shown="\"Tune\"" w509 {
              frame "Checklist", Default {
              }
              frame "Tune" {
                n341 = call-poly <vilib>:"NT Read Value.vi"("Default Value"=dbl[] [0.0, 0.0, 0.0, 0.0, 0.0, 0.0], "Name"="Current_Driver_Profile_Setpoints") -> ("Numeric Array"=w600:dbl[])  [unwired: 8 in, 1 out]
                n342 = Array To Cluster(array=w600) -> (cluster=w596:T23)
                "Current_Driver_Profile_Setpoints_GUI" <- w596
                n343 = feedback #4(dbl[] [0.0, 0.0, 0.0, 0.0, 0.0, 0.0] ("Default Value")) -> (w599:dbl[])
                n344 = feedback-in #4(w600) -> ()
                n345 = Not Equal?(x=w600, y=w599) -> (x != y?=w598:bool[])
                n346 = Or Array Elements(Boolean array=w598) -> (logical OR=w597:bool)
                n347 = case shown="True" w597 {
                  tunnel: w596 -> [_ w604]
                  frame False {
                  }
                  frame True {
                    n348 = property on="New_Driver_Profile_Setpoints_GUI" class="Clust (strict)"("Value"=w604) -> ()  [unwired: 2 in, 2 out]
                  }
                }
              }
            }
            n349 = local read "Legal_Drivers_GUI"() -> (w584:string[])
            n350 = local read "Driver Profile (1)"() -> (w583:u16)
            n351 = Cluster To Array(cluster="New_Driver_Profile_Setpoints_GUI") -> (array=w513:dbl[])
            n352 = And(x="Calibrate_Wheels_GUI", y="Arm_Calibrate_Wheels_GUI") -> (x .and. y?=w516:bool)
            n353 = Not(x="Arm_Calibrate_Wheels_GUI") -> (.not. x?=w591:bool)
            n354 = To Long Integer(number=w583) -> (32bit integer=w581:i32)
            n355 = call "ReducedBWSendToNT.vim"("Value In"="Home_Wheels_GUI", "NT Name"="Home_Wheels" ("Name")) -> ()  [unwired: 1 out]
            n356 = Index Array(array=w584, index=w581) -> (element=→"Current_Driver_Profile_GUI":string)
            n357 = call "ReducedBWSendToNT.vim"("Value In"="Apply_Driver_Profile_Setpoints_GUI", "NT Name"="Apply_Driver_Profile_Setpoints" ("Name")) -> ()  [unwired: 1 out]
            n358 = call "ReducedBWSendToNT.vim"("Value In"=w513, "NT Name"="New_Driver_Profile_Setpoints" ("Name")) -> ()  [unwired: 1 out]
            n359 = call "ReducedBWSendToNT.vim"("Value In"=w516, "NT Name"="Calibrate_Wheels" ("Name")) -> ()  [unwired: 1 out]
            n360 = Select(t=cluster{u32, u32}[] [{11776947, 16448250}, {16448250, 16448250}] ("Colors [4]"), s=w591, f=cluster{u32, u32}[] [{6618880, 16448250}, {16448250, 16448250}] ("Colors [4]")) -> (s? t:f=w590:cluster{u32, u32}[])
            n361 = property on="Calibrate_Wheels_GUI" class="Bool"("Colors [4]"=w590) -> ()  [unwired: 2 in, 2 out]
          }
          frame #7 {
            # "climber subsystem"
            # "ball handling subsystems"
            # "ball handling and climbing subsystems"
            n362 = local read "Dashboard Tab"() -> (w605:T1)
            n363 = case shown="\"Tune\"" w605 {
              frame "Checklist", Default {
              }
              frame "Tune" {
                n364 = call-poly <vilib>:"NT Read Value.vi"("Default Value"="UNKNOWN", "Name"="Color_Sensor_Reading") -> ("String"=→"Color_Sensor_Reading_GUI":string)  [unwired: 8 in, 1 out]
                n365 = call-poly <vilib>:"NT Read Value.vi"("Name"="Climber_Active_Arm_Position") -> ("Numeric"=→"Climber_Active_Arm_Position_GUI":dbl)  [unwired: 9 in, 1 out]
              }
            }
            n366 = call-poly <vilib>:"NT Read Value.vi"("Name"="Current_Balls") -> ("Numeric"=w609:dbl)  [unwired: 9 in, 1 out]
            n367 = call-poly <vilib>:"NT Read Value.vi"("Name"="Intake_Motor_Failure_Left") -> ("Boolean"=→"Intake_Motor_Failure_Left_GUI":bool)  [unwired: 9 in, 1 out]
            n368 = call-poly <vilib>:"NT Read Value.vi"("Name"="Indexer_Beam_Break") -> ("Boolean"=→"Indexer_Beam_Break_GUI":bool)  [unwired: 9 in, 1 out]
            n369 = call-poly <vilib>:"NT Read Value.vi"("Name"="Tower_Beam_Break") -> ("Boolean"=→"Tower_Beam_Break_GUI":bool)  [unwired: 9 in, 1 out]
            n370 = call-poly <vilib>:"NT Read Value.vi"("Name"="Intake_Intaking") -> ("Boolean"=→"Intake_Intaking_GUI":bool)  [unwired: 9 in, 1 out]
            n371 = call-poly <vilib>:"NT Read Value.vi"("Name"="Intake_Motor_Failure_Right") -> ("Boolean"=→"Intake_Motor_Failure_Right_GUI":bool)  [unwired: 9 in, 1 out]
            n372 = To Long Integer(number=w609) -> (32bit integer=→"Current_Balls_GUI":i32)
            n373 = call-poly <vilib>:"NT Read Value.vi"("Name"="Climber_Climbing") -> ("Boolean"=→"Climber_Climbing_GUI":bool)  [unwired: 9 in, 1 out]
          }
          frame #8 {
            # "shooter and turret subsystems"
            n374 = local read "Dashboard Tab"() -> (w626:T1)
            n375 = case shown="\"Tune\"" w626 {
              frame "Checklist", Default {
              }
              frame "Tune" {
                n376 = call-poly <vilib>:"NT Read Value.vi"("Name"="Kicker_Temperature") -> ("Numeric"=→"Kicker_Temperature_GUI":dbl)  [unwired: 9 in, 1 out]
                n377 = call-poly <vilib>:"NT Read Value.vi"("Name"="Kicker_Speed") -> ("Numeric"=→"Kicker_Speed_GUI":dbl)  [unwired: 9 in, 1 out]
                n378 = call-poly <vilib>:"NT Read Value.vi"("Name"="Shooter_Upper_Temperature") -> ("Numeric"=→"Shooter_Upper_Temperature_GUI":dbl)  [unwired: 9 in, 1 out]
                n379 = call-poly <vilib>:"NT Read Value.vi"("Name"="Shooter_Lower_Speed") -> ("Numeric"=→"Shooter_Lower_Speed_GUI":dbl)  [unwired: 9 in, 1 out]
                n380 = call-poly <vilib>:"NT Read Value.vi"("Name"="Shooter_Upper_Speed") -> ("Numeric"=→"Shooter_Upper_Speed_GUI":dbl)  [unwired: 9 in, 1 out]
                n381 = call-poly <vilib>:"NT Read Value.vi"("Name"="Shooter_Lower_Temperature") -> ("Numeric"=→"Shooter_Lower_Temperature_GUI":dbl)  [unwired: 9 in, 1 out]
                n382 = call-poly <vilib>:"NT Read Value.vi"("Name"="Turret_Limit_A") -> ("Boolean"=→"Turret_Limit_A_GUI":bool)  [unwired: 9 in, 1 out]
                n383 = call-poly <vilib>:"NT Read Value.vi"("Name"="Cowl_Limit_A") -> ("Boolean"=→"Cowl_Limit_A_GUI":bool)  [unwired: 9 in, 1 out]
                n384 = call-poly <vilib>:"NT Read Value.vi"("Name"="Turret_Limit_B") -> ("Boolean"=→"Turret_Limit_B_GUI":bool)  [unwired: 9 in, 1 out]
                n385 = call-poly <vilib>:"NT Read Value.vi"("Name"="Turret_Angle") -> ("Numeric"=→"Turret_Angle_GUI":dbl)  [unwired: 9 in, 1 out]
                n386 = call-poly <vilib>:"NT Read Value.vi"("Name"="Cowl_Angle") -> ("Numeric"=→"Cowl_Angle_GUI":dbl)  [unwired: 9 in, 1 out]
              }
            }
            n387 = call-poly <vilib>:"NT Read Value.vi"("Name"="Shooter_Spinning") -> ("Boolean"=→"Shooter_Spinning_GUI":bool)  [unwired: 9 in, 1 out]
            n388 = call-poly <vilib>:"NT Read Value.vi"("Name"="Shooter_Firing") -> ("Boolean"=→"Shooter_Firing_GUI":bool)  [unwired: 9 in, 1 out]
            n389 = call-poly <vilib>:"NT Read Value.vi"("Name"="Pointed_At_Target") -> ("Boolean"=→"Pointed_At_Target_GUI":bool)  [unwired: 9 in, 1 out]
            n390 = call-poly <vilib>:"NT Read Value.vi"("Name"="Shooter_Ready") -> ("Boolean"=→"Shooter_Ready_GUI":bool)  [unwired: 9 in, 1 out]
            n391 = call "ReducedBWSendToNT.vim"("Value In"="Home_Turret_GUI", "NT Name"="Home_Turret" ("Name")) -> ()  [unwired: 1 out]
            n392 = call "ReducedBWSendToNT.vim"("Value In"="Home_Cowl_GUI", "NT Name"="Home_Cowl" ("Name")) -> ()  [unwired: 1 out]
            n393 = call-poly <vilib>:"NT Read Value.vi"("Name"="Shooter_Lower_Overheating") -> ("Boolean"=w676:bool)  [unwired: 9 in, 1 out]
            "Shooter_Lower_Overheating_GUI" <- w676
            n394 = call-poly <vilib>:"NT Read Value.vi"("Name"="Shooter_Upper_Overheating") -> ("Boolean"=w675:bool)  [unwired: 9 in, 1 out]
            "Shooter_Upper_Overheating_GUI" <- w675
            n395 = call-poly <vilib>:"NT Read Value.vi"("Name"="Kicker_Overheating") -> ("Boolean"=w651:bool)  [unwired: 9 in, 1 out]
            "Kicker_Overheating_GUI" <- w651
            n396 = Select(t=u32 16711680 ("Numeric Text.Text Colors:Text Color"), s=w676, f=u32 4934475 ("Numeric Text.Text Colors:Text Color")) -> (s? t:f=w709:u32)
            n397 = Select(t=u32 16711680 ("Numeric Text.Text Colors:Text Color"), s=w675, f=u32 4934475 ("Numeric Text.Text Colors:Text Color")) -> (s? t:f=w710:u32)
            n398 = Select(t=u32 16711680 ("Numeric Text.Text Colors:Text Color"), s=w651, f=u32 4934475 ("Numeric Text.Text Colors:Text Color")) -> (s? t:f=w655:u32)
            n399 = property on="Shooter_Lower_Temperature_GUI" class="DigNum (strict)"("NumText.BG Color"=w709) -> ()  [unwired: 2 in, 2 out]
            n400 = property on="Shooter_Upper_Temperature_GUI" class="DigNum (strict)"("NumText.BG Color"=w710) -> ()  [unwired: 2 in, 2 out]
            n401 = property on="Kicker_Temperature_GUI" class="DigNum (strict)"("NumText.BG Color"=w655) -> ()  [unwired: 2 in, 2 out]
            n402 = call "ReducedBWSendToNT.vim"("Value In"="Apply_Firing_Delay_GUI", "NT Name"="Apply_Firing_Delay" ("Name")) -> ()  [unwired: 1 out]
            n403 = call "ReducedBWSendToNT.vim"("Value In"="New_Firing_Delay_GUI", "NT Name"="New_Firing_Delay" ("Name")) -> ()  [unwired: 1 out]
            n404 = call "ReducedBWSendToNT.vim"("Value In"="Apply_Radial_Firing_Delay_GUI", "NT Name"="Apply_Radial_Firing_Delay" ("Name")) -> ()  [unwired: 1 out]
            n405 = call "ReducedBWSendToNT.vim"("Value In"="New_Radial_Firing_Delay_GUI", "NT Name"="New_Radial_Firing_Delay" ("Name")) -> ()  [unwired: 1 out]
            n406 = Build Array("N/A") -> (w696:string[])
            n407 = To Double Precision Float(number="Selected_Shooter_Setpoint_Index") -> (double precision float=w669:dbl)
            n408 = call-poly <vilib>:"NT Read Value.vi"("Default Value"=w696, "Name"="Legal_Shooter_Setpoints") -> ("String Array"=w695:string[])  [unwired: 8 in, 1 out]
            n409 = call "ReducedBWSendToNT.vim"("Value In"="New_Shooter_Setpoint_Turret_GUI", "NT Name"="New_Shooter_Setpoint_Turret" ("Name")) -> ()  [unwired: 1 out]
            n410 = call-poly <vilib>:"NT Read Value.vi"("Name"="Selected_Shooter_Setpoint_Turret_Value") -> ("Numeric"=w641:dbl)  [unwired: 9 in, 1 out]
            "Selected_Shooter_Setpoint_Turret_Value_GUI" <- w641
            n411 = call-poly <vilib>:"NT Read Value.vi"("Default Value"=0.0, "Name"="Selected_Firing_Delay") -> ("Numeric"=w647:dbl)  [unwired: 8 in, 1 out]
            "Selected_Firing_Delay_GUI" <- w647
            n412 = call "ReducedBWSendToNT.vim"("Value In"="New_Shooter_Setpoint_Angle_GUI", "NT Name"="New_Shooter_Setpoint_Angle" ("Name")) -> ()  [unwired: 1 out]
            n413 = call "ReducedBWSendToNT.vim"("Value In"="Apply_New_Shooter_Setpoint_GUI", "NT Name"="Apply_New_Shooter_Setpoint" ("Name")) -> ()  [unwired: 1 out]
            n414 = call-poly <vilib>:"NT Read Value.vi"("Default Value"=0.0, "Name"="Selected_Radial_Firing_Delay") -> ("Numeric"=w627:dbl)  [unwired: 8 in, 1 out]
            "Selected_Radial_Firing_Delay_GUI" <- w627
            n415 = call-poly <vilib>:"NT Read Value.vi"("Name"="Selected_Shooter_Setpoint_Angle_Value") -> ("Numeric"=w678:dbl)  [unwired: 9 in, 1 out]
            "Selected_Shooter_Setpoint_Angle_Value_GUI" <- w678
            n416 = call "ReducedBWSendToNT.vim"("Value In"=w669, "NT Name"="Selected_Shooter_Setpoint_Index" ("Name")) -> ()  [unwired: 1 out]
            n417 = call-poly <vilib>:"NT Read Value.vi"("Name"="Selected_Shooter_Setpoint_Ratio_Value") -> ("Numeric"=w683:dbl)  [unwired: 9 in, 1 out]
            "Selected_Shooter_Setpoint_Ratio_Value_GUI" <- w683
            n418 = call "ReducedBWSendToNT.vim"("Value In"="New_Shooter_Setpoint_Ratio_GUI", "NT Name"="New_Shooter_Setpoint_Ratio" ("Name")) -> ()  [unwired: 1 out]
            n419 = property on="Selected_Shooter_Setpoint_Index" class="Ring (strict)"("Strings []"=w695) -> ()  [unwired: 2 in, 2 out]
            n420 = call "ReducedBWSendToNT.vim"("Value In"="New_Shooter_Setpoint_Speed_GUI", "NT Name"="New_Shooter_Setpoint_Speed" ("Name")) -> ()  [unwired: 1 out]
            n421 = call-poly <vilib>:"NT Read Value.vi"("Name"="Selected_Shooter_Setpoint_Speed_Value") -> ("Numeric"=w689:dbl)  [unwired: 9 in, 1 out]
            "Selected_Shooter_Setpoint_Speed_Value_GUI" <- w689
            n422 = feedback #5(0.0 ("Numeric")) -> (w643:dbl)
            n423 = feedback-in #5(w641) -> ()
            n424 = feedback #6(0.0 ("Numeric")) -> (w680:dbl)
            n425 = feedback-in #6(w678) -> ()
            n426 = feedback #7(0.0 ("Numeric")) -> (w649:dbl)
            n427 = feedback-in #7(w647) -> ()
            n428 = feedback #8(0.0 ("Numeric")) -> (w685:dbl)
            n429 = feedback-in #8(w683) -> ()
            n430 = feedback #9(0.0 ("Numeric")) -> (w633:dbl)
            n431 = feedback-in #9(w627) -> ()
            n432 = feedback-in #10(w689) -> ()
            n433 = feedback #10(0.0 ("Numeric")) -> (w690:dbl)
            n434 = Not Equal?(x=w643, y=w641) -> (x != y?=w642:bool)
            n435 = Not Equal?(x=w680, y=w678) -> (x != y?=w679:bool)
            n436 = Not Equal?(x=w685, y=w683) -> (x != y?=w684:bool)
            n437 = Not Equal?(x=w647, y=w649) -> (x != y?=w650:bool)
            n438 = Not Equal?(x=w627, y=w633) -> (x != y?=w630:bool)
            n439 = Not Equal?(x=w690, y=w689) -> (x != y?=w688:bool)
            n440 = case shown="True" w642 {
              tunnel: w641 -> [_ w736]
              frame False {
              }
              frame True {
                n441 = property on="New_Shooter_Setpoint_Turret_GUI" class="DigNum (strict)"("Value"=w736) -> ()  [unwired: 2 in, 2 out]
              }
            }
            n442 = case shown="True" w650 {
              tunnel: w647 -> [_ w737]
              frame False {
              }
              frame True {
                n443 = property on="New_Firing_Delay_GUI" class="DigNum (strict)"("Value"=w737) -> ()  [unwired: 2 in, 2 out]
              }
            }
            n444 = case shown="True" w679 {
              tunnel: w678 -> [_ w738]
              frame False {
              }
              frame True {
                n445 = property on="New_Shooter_Setpoint_Angle_GUI" class="DigNum (strict)"("Value"=w738) -> ()  [unwired: 2 in, 2 out]
              }
            }
            n446 = case shown="True" w684 {
              tunnel: w683 -> [_ w739]
              frame False {
              }
              frame True {
                n447 = property on="New_Shooter_Setpoint_Ratio_GUI" class="DigNum (strict)"("Value"=w739) -> ()  [unwired: 2 in, 2 out]
              }
            }
            n448 = case shown="True" w630 {
              tunnel: w627 -> [_ w735]
              frame False {
              }
              frame True {
                n449 = property on="New_Radial_Firing_Delay_GUI" class="DigNum (strict)"("Value"=w735) -> ()  [unwired: 2 in, 2 out]
              }
            }
            n450 = call "ReducedBWSendToNT.vim"("Value In"="Targeting_Override_GUI", "NT Name"="Override_Targeting_Decisions" ("Name")) -> ()  [unwired: 1 out]
            n451 = case shown="True" w688 {
              tunnel: w689 -> [_ w740]
              frame False {
              }
              frame True {
                n452 = property on="New_Shooter_Setpoint_Speed_GUI" class="DigNum (strict)"("Value"=w740) -> ()  [unwired: 2 in, 2 out]
              }
            }
          }
          frame #9 {
            w768 = FALSE  # wide angle camera
            # "manage targeting reticules"
            # "manage audible warnings"
            # "error management and driver assistance"
            n453 = local read "Shooter_Lower_Overheating_GUI"() -> (w785:bool)
            n454 = local read "Intake_Motor_Failure_Right_GUI"() -> (w793:bool)
            n455 = local read "Shooter_Upper_Overheating_GUI"() -> (w784:bool)
            n456 = local read "Intake_Motor_Failure_Left_GUI"() -> (w790:bool)
            n457 = local read "Swerve_Azimuth_Fault_Array"() -> (w773:bool[])
            n458 = local read "Swerve_Shifter_Failure_Array"() -> (w796:bool[])
            n459 = local read "Swerve_Overheating_Array"() -> (w774:bool[])
            n460 = local read "Kicker_Overheating_GUI"() -> (w748:bool)
            n461 = local read "Battery_Critical_GUI"() -> (w805:bool)
            n462 = local read "Compressor_On_GUI"() -> (w778:bool)
            n463 = local read "Vision_Fault_GUI"() -> (w780:bool)
            n464 = local read "IMU_Failure_GUI"() -> (w803:bool)
            n465 = Initialize Array(FALSE ("element"), 26 ("dimension size")) -> (w766:bool[])
            n466 = Initialize Array(FALSE ("element"), 26 ("dimension size")) -> (w764:bool[])
            n467 = Replace Array Subset(array=w766, new element=w778, index=4) -> (w776:bool[])
            n468 = Replace Array Subset(array=w776, new element=w768, index=25) -> (w762:bool[])
            n469 = Replace Array Subset(array=w762, new element=w805, index=0) -> (w763:bool[])
            n470 = Initialize Array(FALSE, 26 ("dimension size")) -> (w823:bool[])
            n471 = Or Array Elements(Boolean array=w796) -> (logical OR=→"Swerve_Shifter_Failure":bool)
            n472 = Or Array Elements(Boolean array=w773) -> (logical OR=→"Swerve_Azimuth_Fault":bool)
            n473 = Or Array Elements(Boolean array=w774) -> (logical OR=→"Swerve_Overheating":bool)
            n474 = Replace Array Subset(array=w764, new element=w803, index=7) -> (w801:bool[])
            n475 = Replace Array Subset(array=w801, new element=w773, index=8) -> (w799:bool[])
            n476 = Replace Array Subset(array=w799, new element=w774, index=12) -> (w797:bool[])
            n477 = Replace Array Subset(array=w797, new element=w796, index=16) -> (w794:bool[])
            n478 = Replace Array Subset(array=w794, new element=w793, index=20) -> (w791:bool[])
            n479 = Replace Array Subset(array=w791, new element=w790, index=22) -> (w788:bool[])
            n480 = Replace Array Subset(array=w788, new element=w785, index=23) -> (w786:bool[])
            n481 = Replace Array Subset(array=w786, new element=w784, index=24) -> (w767:bool[])
            n482 = Replace Array Subset(array=w767, new element=w780, index=3) -> (w751:bool[])
            n483 = Replace Array Subset(array=w751, new element=w748, index=21) -> (w750:bool[])
            n484 = Build Array("Error_Help", "Driver_Help", "Manipulator_Help") -> (w813:bool[])
            n485 = Or Array Elements(Boolean array=w813) -> (logical OR=w765:bool)
            n486 = Not(x=w765) -> (.not. x?=w826:bool)
            n487 = Build Array (concatenate)(w826, w813) -> (w825:bool[])
            n488 = property on="Help Graphic" class="ImageControl"("Visible"=w765) -> ()  [unwired: 2 in, 2 out]
            n489 = call "StateSelection.vi"("Disallowed States"=bool[] [FALSE, FALSE, FALSE, FALSE], "State Triggers"=w825, "State Names"=string[] ["No Help", "Error Help", "Driver Help", "Manipulator Help"]) -> ("Selected State"=w831:string)
            n490 = case shown="\"Error Help\"" w831 {
              tunnel: [_ w861 w862 w864] -> w775
              tunnel: w823 -> [_ w859 _ _]
              tunnel: w763 -> [_ w858 _ _]
              tunnel: w750 -> [_ w860 _ _]
              tunnel: w765 -> [_ w857 _ _]
              frame "No Help", Default {
              }
              frame "Error Help" {
                n491 = call "RenderRobotSystemsDiagram.vi"("Enable"=w857, "Cautions"=w858, "Nominals"=w859, "Alarms"=w860) -> ("Robot Systems Diagram"=w861:T3)  [unwired: 1 in]
              }
              frame "Driver Help" {
                n492 = call "RenderJoystickDiagram.vi"("Joystick Graphic Filename"="driver joystick diagram.png") -> ("Image Out"=w862:T3)  [unwired: 10 in]
              }
              frame "Manipulator Help" {
                n493 = call "RenderJoystickDiagram.vi"("Joystick Graphic Filename"="manipulator joystick diagram.png") -> ("Image Out"=w864:T3)  [unwired: 10 in]
              }
            }
            "Help Graphic" <- w775
            n494 = Or Array Elements(Boolean array=w813) -> (logical OR=w815:bool)
            n495 = Not(x=w815) -> (.not. x?=w814:bool)
            n496 = Or(x=w814, y=w813) -> (x .or. y?=w812:bool[])
            n497 = Index Array(array=w812, index #1=0 ("index")) -> (element #1=w818:bool, element #2=w817:bool, element #3=w816:bool)  [unwired: 2 in]
            n498 = Select(t=T16."Enabled" ("Disabled"), s=w816, f=T16."Disabled and Grayed Out" ("Disabled")) -> (s? t:f=w820:T16)
            n499 = Select(t=T16."Enabled" ("Disabled"), s=w818, f=T16."Disabled and Grayed Out" ("Disabled")) -> (s? t:f=w855:T16)
            n500 = Select(t=T16."Enabled" ("Disabled"), s=w817, f=T16."Disabled and Grayed Out" ("Disabled")) -> (s? t:f=w856:T16)
            n501 = property on="Error_Help" class="Bool (strict)"("DisabledEnum"=w855) -> ()  [unwired: 2 in, 2 out]
            n502 = property on="Driver_Help" class="Bool (strict)"("DisabledEnum"=w856) -> ()  [unwired: 2 in, 2 out]
            n503 = property on="Manipulator_Help" class="Bool (strict)"("DisabledEnum"=w820) -> ()  [unwired: 2 in, 2 out]
            n504 = First Call?() -> (First Call?: T/F=w747:bool)
            n505 = call-poly <vilib>:"NT Read Value.vi"("Default Value"=FALSE, "Name"="Master_Alarm") -> ("Boolean"=w743:bool)  [unwired: 8 in, 1 out]
            n506 = call "Timer.vi"("Reset Timer"=w747) -> ("Time (ms)"=w746:u32)
            n507 = Greater?(x=w746, y=u32 2500) -> (0:w744:bool)
            n508 = local read "Arm_Calibrate_Wheels_GUI"() -> (w753:bool)
            n509 = local read "Arm_Calibrate_Joysticks"() -> (w754:bool)
            n510 = call-poly <vilib>:"NT Read Value.vi"("Default Value"=0.0, "Name"="Number_of_Master_Alarms") -> ("Numeric"=w757:dbl)  [unwired: 8 in, 1 out]
            n511 = And(x=w744, y=w743) -> (x .and. y?=w742:bool)
            n512 = To Long Integer(number=w757) -> (32bit integer=w756:i32)
            n513 = call "EdgeTrigger.vi"("Input Signal"="Mute_Audible_Warnings") -> ("Rising Edge Trigger"=w839:bool)  [unwired: 2 out]
            n514 = call "BlinkLight.vi"() -> ("Blinked"=w844:bool)  [unwired: 1 in]
            n515 = local read "No_Secondary_Camera"() -> (w769:bool)
            n516 = Number To Decimal String(number=w756) -> (decimal integer string=w845:string)  [unwired: 1 in]
            n517 = local read "Intake_Intaking_GUI"() -> (w772:bool)
            n518 = feedback #11(TRUE ("t")) -> (w837:bool)
            n519 = Not(x=w837) -> (.not. x?=w836:bool)
            n520 = Select(t=w836, s=w839, f=w837) -> (s? t:f=w741:bool)
            "Audible_Warnings_Enabled_GUI" <- w741
            n521 = feedback-in #11(w741) -> ()
            n522 = Select(t=w844, s=w742, f=FALSE) -> (s? t:f=w848:bool)
            "Master_Caution_GUI_1" <- w848
            "Master_Caution_GUI_0" <- w848
            "Master_Caution_GUI_2" <- w848
            n523 = Concatenate Strings("MASTER ALARM (" ("string"), w845, ")" ("string")) -> (w846:string)
            n524 = Select(t=w846, s=w848, f="") -> (s? t:f=w847:string)
            n525 = Compound Arithmetic op=OR(w754, w753) -> (w752:bool)
            n526 = Not(x=w769) -> (.not. x?=w770:bool)
            n527 = call "ReducedBWSendToNT.vim"("Value In"=w752, "NT Name"="Some_Switch_Armed" ("Name")) -> ()  [unwired: 1 out]
            n528 = property on="Master_Caution_GUI_0" class="Bool (strict)"("BoolText.Text"=w847) -> ()  [unwired: 2 in, 2 out]
            n529 = property on="Master_Caution_GUI_1" class="Bool (strict)"("BoolText.Text"=w847) -> ()  [unwired: 2 in, 2 out]
            n530 = property on="Master_Caution_GUI_2" class="Bool (strict)"("BoolText.Text"=w847) -> ()  [unwired: 2 in, 2 out]
            n531 = And(x=w770, y=w772) -> (x .and. y?=→"CARGO_Ret_Left" →"CARGO_Ret_Right":bool)
            n532 = Select(t=cluster{u32, u32}[] [{6618880, 16448250}, {16448250, 16448250}] ("Colors [4]"), s=w741, f=cluster{u32, u32}[] [{16755474, 16448250}, {16448250, 16448250}] ("Colors [4]")) -> (s? t:f=w835:cluster{u32, u32}[])
            n533 = property on="Mute_Audible_Warnings" class="Bool"("Colors [4]"=w835) -> ()  [unwired: 2 in, 2 out]
          }
          frame #10 {
            # "flush NT tables"
            n534 = call <vilib>:"NT Flush Data Updates.vi"() -> ()  [unwired: 11 in, 1 out]
          }
        }
      }
    }
  }
  n535 = call "InitChecklistCustom.vi"("ListBox in"=w3) -> ()  [unwired: 1 in]
  n536 = control-ref of="Command Params"() -> (w13:refnum<vi>)
  n537 = while {
    tunnel: [w873] -> _
    tunnel: w29 -> [w872]
    tunnel: w28 -> [_]
    tunnel: w24 -> [w871]
    tunnel: w14 -> [w870]
    tunnel: w13 -> [w869]
    shift-right: [w868] -> _
    shift-left: _ -> [w867]
    tunnel: w12 -> [w866]
    i -> [w873]
    stop <- FALSE stop-if-true
    n538 = event shown="[4] \"CheckList\": Double Click" {
      selector: w872 -> [_ _ _ _ _ _ _ _]
      dyn-events: _ -> [_ _ _ _ _ _ _ _]
      timeout: u32 60 ("milliseconds to wait") -> [_ _ _ _ _ _ _ _]
      tunnel: w871 -> [_ _ _ _ _ _ _ _]
      tunnel: w870 -> [_ _ _ _ _ _ _ _]
      tunnel: w869 -> [w879 w920 _ _ _ _ _ _]
      tunnel: [w878 w918 w927 w937 w944 w956 w968 w981] -> w868
      tunnel: w867 -> [w878 w918 _ _ w944 w956 w968 w981]
      tunnel: w866 -> [w876 _ _ _ _ _ _ _]
      event Timeout {
        n539 = event-data() -> ()  [unwired: 1 in, 1 out]
        n540 = local read "Mode"() -> (w881:T7)
        n541 = case shown="\"TeleOp\", Default" "Dashboard Tab" {
          tunnel: "TestMode/Automatic/" ("Name Pattern") -> [_ _ w893 _ _]
          tunnel: T24 [{"Operation"=enum."Clear", "Color Box"=14013909}, {"Operation"=enum."Clear", "Color Box"=14013909}, {"Operation"=enum."Clear", "Color Box"=14013909}, {"Operation"=enum."Clear", "Color Box"=14013909}, {"Operation"=enum."Update", "Color Box"=14013909}, {"Operation"=enum."Update", "Color Box"=16777215}, {"Operation"=enum."Clear", "Color Box"=14013909}, {"Operation"=enum."Clear", "Color Box"=14013909}, {"Operation"=enum."Clear", "Color Box"=14013909}] -> [_ _ w890 _ w912]
          tunnel: w881 -> [_ _ w889 _ w911]
          tunnel: u32[] [15790320, 15790320, 15790320, 15790320, 16777215, 16777215, 15790320, 15790320, 15790320] -> [_ _ _ _ w917]
          tunnel: w879 -> [_ _ _ _ w905]
          tunnel: w876 -> [_ _ _ _ _]
          frame "TeleOp", Default {
          }
          frame "Tune" {
          }
          frame "Test" {
            n542 = Index Array(array=w890, index=w889) -> (element=w891:T26)
            n543 = Unbundle(w891) -> ("Operation"=w892:enum16{"Update", "Clear"})  [unwired: 1 out]
            n544 = call <vilib>:"NT Read String.vi"("Name"="TestMode/TestName") -> ("String"=w887:string)  [unwired: 9 in, 1 out]
            n545 = call <vilib>:"NT Read and Format Entries as Tree.vi"("Operation"=w892, "Name Pattern"=w893) -> ()  [unwired: 8 in, 2 out]
            n546 = case shown="\"\"" w887 {
              tunnel: "TestMode/TestProgress" ("Name") -> [w895 _]
              tunnel: "TestMode/TestProgressText" ("Name") -> [w894 _]
              frame Default {
                n547 = call <vilib>:"NT Read Number.vi"("Name"=w895) -> ("Numeric"=w896:dbl)  [unwired: 9 in, 1 out]
                n548 = call <vilib>:"NT Read String.vi"("Name"=w894) -> ("String"=w897:string)  [unwired: 9 in, 1 out]
                n549 = Bundle("Numeric"=w896, "String"=w897) -> (→"Progress":cluster{"Numeric":dbl, "String":string})  [unwired: 1 in]
              }
              frame "" {
                n550 = property on="Progress" class="Clust (strict)"("Visible"=FALSE) -> ()  [unwired: 2 in, 2 out]
              }
            }
          }
          frame "Variables" {
            w902 = string[] ["CameraPublisher", "Usage", "DB"]  # Items to initially close
            n551 = First Call?() -> (First Call?: T/F=w903:bool)
            n552 = control-ref of="Tree"() -> (w904:refnum<vi>)
            n553 = Select(t=w902, s=w903, f=string[] []) -> (s? t:f=w900:string[])
            n554 = call <vilib>:"NT Read and Format Entries as Tree.vi"("Tags to  Close"=w900, "Tree Refnum"=w904) -> ()  [unwired: 8 in, 2 out]
          }
          frame "Commands" {
            w913 = u32 5789784 ("Color Box")
            w914 = T27 {"Row"=-1, "Column"=-2} ("Active Cell:Active Cell")
            w916 = T27 {"Row"=-2, "Column"=-2} ("Active Cell:Active Cell")
            n555 = Index Array(array=w917, index=w911) -> (element=w915:u32)
            n556 = Index Array(array=w912, index=w911) -> (element=w910:T26)
            n557 = Unbundle(w910) -> ("Operation"=w909:enum16{"Update", "Clear"})  [unwired: 1 out]
            n558 = local read "Command Selection"() -> (w908:i32)
            n559 = property on="Command Selection" class="MCListbox (strict)"("ActiveCell"=w916, "CellBG"=w915, "ActiveCell"=w914, "CellBG"=w913) -> ()  [unwired: 2 in, 2 out]
            n560 = call <vilib>:"WPI_DashboardUpdate RPC Info.vi"("Operation"=w909) -> ("update"=w907:bool, "commands"=w906:string[][])  [unwired: 9 in]
            n561 = property on="Command Selection" class="MCListbox (strict)"("ItemNames"=w906) -> ()  [unwired: 2 in, 2 out]
            n562 = property on="Command Params" class="Tbl (strict)"("Active Cell"=w916, "Cell BG Color"=w915, "Active Cell"=w914, "Cell BG Color"=w913) -> ()  [unwired: 2 in, 2 out]
            n563 = call <vilib>:"WPI_DashboardUpdate Command Params.vi"("Update"=w907, "NewVal"=w908, "Commands"=w906, "Param Tbl"=w905) -> ()  [unwired: 7 in, 1 out]
          }
        }
        n564 = call <vilib>:"Connextion Info.vi"() -> ("Connected"=→"NT Connection":bool)  [unwired: 10 in, 1 out]
      }
      event "Command Selection": Value Change {
        # "Get the params and show in table"
        n565 = event-data() -> ("NewVal"=w921:i32)  [unwired: 1 in]
        n566 = property on="Command Selection" class="MCListbox (strict)"() -> ("ItemNames"=w919:string[][])  [unwired: 2 in, 2 out]
        n567 = call <vilib>:"WPI_DashboardUpdate Command Params.vi"("NewVal"=w921, "Commands"=w919, "Param Tbl"=w920) -> ()  [unwired: 8 in, 1 out]
      }
      event "Execute Command": Value Change {
        # "Started one, Unique ID holds\nresponse"
        n568 = event-data() -> ()  [unwired: 1 in, 1 out]
        n569 = property on="Command Selection" class="MCListbox (strict)"() -> ("ItemNames"=w932:string[][])  [unwired: 2 in, 2 out]
        n570 = Index Array(array=w932, index (row)="Command Selection", index (col)=0) -> (element=w930:string)
        n571 = call <vilib>:"Invoke Commands.vi"("Command Params"="Command Params", "Function Name"=w930) -> ("Params"=w926:u8, "Started"=w925:bool)  [unwired: 7 in, 1 out]
        n572 = Array Subset(array="Command Params", length (row)=w926) -> (w927:string[][])  [unwired: 3 in]
        n573 = Select(t="Executing" ("Cmd Status"), s=w925, f="" ("Cmd Status")) -> (s? t:f=→"Cmd Status":string)
      }
      event "Command Selection": Double Click {
        n574 = event-data() -> ("Row"=w940:i32)  [unwired: 1 in]
        n575 = property on="Command Selection" class="MCListbox (strict)"() -> ("ItemNames"=w943:string[][])  [unwired: 2 in, 2 out]
        n576 = local read "Command Params"() -> (w939:string[][])
        n577 = Index Array(array=w943, index (row)=w940, index (col)=0) -> (element=w941:string)
        n578 = call <vilib>:"Invoke Commands.vi"("Command Params"=w939, "Function Name"=w941) -> ("Params"=w938:u8, "Started"=w933:bool)  [unwired: 7 in, 1 out]
        n579 = Array Subset(array=w939, length (row)=w938) -> (w937:string[][])  [unwired: 3 in]
        n580 = Select(t="Executing" ("Cmd Status"), s=w933, f="" ("Cmd Status")) -> (s? t:f=w934:string)
        n581 = local write "Cmd Status"(w934) -> ()
      }
      event "CheckList": Double Click {
        # "Shift clears all"
        # "Update symbols on the listbox"
        n582 = event-data() -> ("PlatMods.Shift"=w945:bool, "Row"=w947:i32)  [unwired: 1 in]
        n583 = case shown="True" w945 {
          tunnel: w947 -> [w951 _]
          tunnel: 1 -> [w950 _]
          frame False {
            n584 = property on="CheckList" class="LstBox (strict)"() -> ("Item Symbols"=w949:i32[])  [unwired: 2 in, 2 out]
            n585 = Replace Array Subset(array=w949, new element=w950, index=w951) -> (w948:i32[])
            n586 = property on="CheckList" class="LstBox (strict)"("Item Symbols"=w948) -> ()  [unwired: 2 in, 2 out]
          }
          frame True {
            w952 = 0 ("Top Row")
            n587 = property on="CheckList" class="LstBox (strict)"() -> ("Number of Rows"=w954:u32)  [unwired: 2 in, 2 out]
            n588 = Initialize Array(0, w954) -> (w953:i32[])
            n589 = property on="CheckList" class="LstBox (strict)"("Top Row"=w952, "Value"=w952, "Item Symbols"=w953) -> ()  [unwired: 2 in, 2 out]
          }
        }
      }
      event "CheckList": Key Down {
        # "Update symbols on the listbox\nLeft and right keys check and uncheck"
        n590 = event-data() -> ("VKey"=w958:T25)  [unwired: 1 in]
        n591 = case shown="\"Left\", \"Right\"" w958 {
          selector: w958 -> [w963 _]
          tunnel: eventvkey."Left" ("VKey") -> [w961 _]
          frame "Left", "Right" {
            n592 = Equal?(x=w961, y=w963) -> (x = y?=w962:bool)
            n593 = Select(t=0, s=w962, f=1) -> (s? t:f=w964:i32)
            n594 = property on="CheckList" class="LstBox (strict)"() -> ("Item Symbols"=w967:i32[])  [unwired: 2 in, 2 out]
            n595 = Replace Array Subset(array=w967, new element=w964, index="CheckList") -> (w966:i32[])
            n596 = property on="CheckList" class="LstBox (strict)"("Item Symbols"=w966) -> ()  [unwired: 2 in, 2 out]
          }
          frame Default {
          }
        }
      }
      event User Event {
        n597 = event-data() -> ("IDs"=w974:cluster{"RPC field ID":u16, "Unique ID":u16}, "String"=w973:string)  [unwired: 1 in]
        n598 = Bundle("IDs"=w974, "String"=w973) -> (w972:T11)  [unwired: 1 in]
        n599 = call <vilib>:"Retrieve RPC Response.vi"("RPC Response"=w972) -> ("Output"=w970:string[][])  [unwired: 10 in]
        n600 = Build Array (concatenate)(w968, w970) -> (w969:string[][])
        n601 = local write "Command Params"(w969) -> ()
        n602 = local write "Cmd Status"("" ("Cmd Status")) -> ()
      }
      event "Tree": Double Click {
        n603 = event-data() -> ("PlatMods"=w980:T28, "Tag"=w977:string)  [unwired: 1 in]
        n604 = Unbundle(w980) -> ("Shift"=w979:bool)  [unwired: 4 out]
        n605 = String Subset(string=w977, length (rest)=1 ("length (rest)")) -> (substring=w976:string)  [unwired: 1 in]
        n606 = Not(x=w979) -> (.not. x?=w978:bool)
        n607 = case shown="\"/\"" w976 {
          tunnel: w977 -> [_ w983]
          tunnel: w978 -> [_ w982]
          frame Default {
          }
          frame "/" {
            n608 = call <vilib>:"NT Update Persistence.vi"("Persistence"=w982, "Name"=w983) -> ()  [unwired: 9 in, 1 out]
          }
        }
      }
    }
  }
  n609 = local write "Dashboard Tab"(T1."Setup/Auto" ("Dashboard Tab")) -> ()
  n610 = while {
    tunnel: u16 1741 ("timeout ms (25000)") -> [w985]
    stop <- FALSE stop-if-true
    n611 = TCP Create Listener(10:w985) -> (0:w984:errorcluster, 3:w986:refnum<k5>)  [unwired: 4 in, 1 out]
    n612 = case shown="No Error" w984 {
      selector: w984 -> [w988 _]
      tunnel: w986 -> [w989 _]
      frame No Error {
        n613 = while {
          tunnel: w989 -> [w992]
          tunnel: w988 -> [w991]
          stop <- FALSE stop-if-true
          n614 = TCP Wait On Listener(8:w991, 11:w992) -> (0:w993:errorcluster, 4:w994:refnum<k5>)  [unwired: 2 in, 3 out]
          n615 = local write "TCP"(w994) -> ()
          n616 = case shown="Error" w993 {
            frame No Error {
            }
            frame Error {
              n617 = Wait (ms)(milliseconds to wait=u32 1000) -> ()  [unwired: 1 out]
            }
          }
        }
      }
      frame Error {
        n618 = Wait (ms)(milliseconds to wait=u32 1000) -> ()  [unwired: 1 out]
      }
    }
  }
  n619 = local write "Command Selection"(u16 0 ("milliseconds to wait")) -> ()
  n620 = local write "Command Params"(string[][] [] ("Command Params")) -> ()
  n621 = global write "WPI_DashboardLogging Global.vi" "Recording"(enum32{"Stop", "Record", "Playback"}."Stop" ("Rec Mode")) -> ()
  n622 = while {
    tunnel: w8 -> [_]
    stop <- FALSE stop-if-true
    # "Error Message Handling"
    n623 = local read "Shooter_Upper_Overheating_GUI"() -> (w1007:bool)
    n624 = local read "Shooter_Lower_Overheating_GUI"() -> (w1008:bool)
    n625 = property on="Actuator Testing" class="Ring (strict)"() -> ("RingText.Text"=w1046:string)  [unwired: 2 in, 2 out]
    n626 = local read "Kicker_Overheating_GUI"() -> (w997:bool)
    n627 = local read "Intake_Motor_Failure_Left_GUI"() -> (w1004:bool)
    n628 = local read "Intake_Motor_Failure_Right_GUI"() -> (w1059:bool)
    n629 = local read "Master_Safety_Override_1"() -> (w1002:bool)
    n630 = local read "Arm_Calibrate_Wheels_GUI"() -> (w1077:bool)
    n631 = local read "Arm_Calibrate_Joysticks"() -> (w1036:bool)
    n632 = local read "Swerve_Shifter_Failure"() -> (w1027:bool)
    n633 = local read "CAN_Bus_Fault_GUI"() -> (w1033:bool)
    n634 = Wait (ms)(milliseconds to wait=u32 200) -> ()  [unwired: 1 out]
    n635 = local read "Swerve_Azimuth_Fault"() -> (w1081:bool)
    n636 = local read "Home_Wheels_GUI"() -> (w1015:bool)
    n637 = Not Equal?(x=w1046, y="No_Test") -> (x != y?=w1053:bool)
    n638 = local read "Swerve_Overheating"() -> (w1090:bool)
    n639 = local read "Super_Test_Mode_GUI"() -> (w1098:bool)
    n640 = call <vilib>:"Space Constant.vi"() -> ("String"=w1044:string)
    n641 = local read "Auto_Test_Mode_GUI"() -> (w1069:bool)
    n642 = local read "Home_Turret_GUI"() -> (w1014:bool)
    n643 = local read "Electrical_Fault_GUI"() -> (w1041:bool)
    n644 = local read "Vision_Fault_GUI"() -> (w999:bool)
    n645 = local read "Home_Cowl_GUI"() -> (w1013:bool)
    n646 = local read "Pressure_Vent_GUI"() -> (w1086:bool)
    n647 = local read "IMU_Failure_GUI"() -> (w1050:bool)
    n648 = local read "Arm_Climber"() -> (w1062:bool)
    n649 = local read "Auto_Error_GUI"() -> (w1074:bool)
    n650 = Search and Replace String(replace all?=TRUE ("replace all? (F)"), input string=w1046, search string="_", replace string=w1044) -> (result string=w1047:string)  [unwired: 4 in, 3 out]
    n651 = local read "Slow_Loop"() -> (w1093:bool)
    n652 = Compound Arithmetic op=OR(w1008, w1007, w997) -> (w1009:bool)
    n653 = Concatenate Strings("testing " ("string"), w1047) -> (w1056:string)
    n654 = Bundle("homing the wheels", "Home_Wheels_GUI"=w1015, 60.0) -> (w1012:cluster{string, "Home_Wheels_GUI":bool, dbl})  [unwired: 1 in]
    n655 = Bundle("homing the turret", "Home_Turret_GUI"=w1014, 60.0) -> (w1011:cluster{string, "Home_Turret_GUI":bool, dbl})  [unwired: 1 in]
    n656 = Bundle("left intake has failed", "Intake_Motor_Failure_Left_GUI"=w1004, 10.0) -> (w1003:T29)  [unwired: 1 in]
    n657 = Bundle("swerve shifter failure, forced into low gear", "Swerve_Shifter_Failure"=w1027, 600.0) -> (w1026:T30)  [unwired: 1 in]
    n658 = Bundle("Lime Light failure, switch to shooter setpoint", "Vision_Fault_GUI"=w999, 600.0) -> (w998:cluster{string, "Vision_Fault_GUI":bool, dbl})  [unwired: 1 in]
    n659 = Bundle("homing the cowl", "Home_Cowl_GUI"=w1013, 60.0) -> (w1010:cluster{string, "Home_Cowl_GUI":bool, dbl})  [unwired: 1 in]
    n660 = Bundle("safeties disengaged", "Master_Safety_Override_1"=w1002, 10.0) -> (w1102:T31)  [unwired: 1 in]
    n661 = Bundle("super test mode", "Super_Test_Mode_GUI"=w1098, 10.0) -> (w1101:cluster{string, "Super_Test_Mode_GUI":bool, dbl})  [unwired: 1 in]
    n662 = Bundle("control latency too high", "Slow_Loop"=w1093, 60.0) -> (w1094:cluster{string, "Slow_Loop":bool, dbl})  [unwired: 1 in]
    n663 = Bundle("drive train overheating", "Swerve_Overheating"=w1090, 60.0) -> (w1089:cluster{string, "Swerve_Overheating":bool, dbl})  [unwired: 1 in]
    n664 = Bundle("pressure venting", "Pressure_Vent_GUI"=w1086, 600.0) -> (w1085:cluster{string, "Pressure_Vent_GUI":bool, dbl})  [unwired: 1 in]
    n665 = Bundle("swerve azimuth failure", "Swerve_Azimuth_Fault"=w1081, 600.0) -> (w1082:T32)  [unwired: 1 in]
    n666 = Bundle("ready to calibrate swerve modules", "Arm_Calibrate_Wheels_GUI"=w1077, 10.0) -> (w1078:T33)  [unwired: 1 in]
    n667 = Bundle("autonomous play failure", "Auto_Error_GUI"=w1074, 10.0) -> (w1073:cluster{string, "Auto_Error_GUI":bool, dbl})  [unwired: 1 in]
    n668 = Bundle("autonomous test mode", "Auto_Test_Mode_GUI"=w1069, 10.0) -> (w1070:cluster{string, "Auto_Test_Mode_GUI":bool, dbl})  [unwired: 1 in]
    n669 = Bundle("shooter or kicker overheating", w1009, 60.0) -> (w1066:cluster{string, bool, dbl})  [unwired: 1 in]
    n670 = Bundle("climber is armed", "Arm_Climber"=w1062, 10.0) -> (w1063:cluster{string, "Arm_Climber":bool, dbl})  [unwired: 1 in]
    n671 = Bundle("right intake has failed", "Intake_Motor_Failure_Right_GUI"=w1059, 10.0) -> (w1058:T34)  [unwired: 1 in]
    n672 = Bundle(w1056, w1053, 10.0) -> (w1052:cluster{string, bool, dbl})  [unwired: 1 in]
    n673 = Bundle("IMU failure, switch shooter setpoint", "IMU_Failure_GUI"=w1050, 600.0) -> (w1048:cluster{string, "IMU_Failure_GUI":bool, dbl})  [unwired: 1 in]
    n674 = Bundle("electrical bus fault, power down", "Electrical_Fault_GUI"=w1041, 60.0) -> (w1040:T35)  [unwired: 1 in]
    n675 = Bundle("ready to calibrate joysticks, wait ten seconds after pressing calibrate", "Arm_Calibrate_Joysticks"=w1036, 10.0) -> (w1037:T36)  [unwired: 1 in]
    n676 = Bundle("CAN bus fault, check wiring", "CAN_Bus_Fault_GUI"=w1033, 60.0) -> (w1035:cluster{string, "CAN_Bus_Fault_GUI":bool, dbl})  [unwired: 1 in]
    n677 = local read "Audible_Warnings_Enabled_GUI"() -> (w1025:bool)
    n678 = Build Array(w1102, w1101, w1094, w1089, w1085, w1082, w1078, w1073, w1070, w1066, w1063, w1058, w1052, w1048, w1040, w1037, w1035, w1026, w1012, w1011, w1010, w1003, w998) -> (w1100:cluster{string, "Vision_Fault_GUI":bool, dbl}[])
    n679 = call "EdgeTrigger.vi"("Input Signal"=w1025) -> ("All Edge Trigger"=w1024:bool)  [unwired: 2 out]
    n680 = call "ErrorMessageBuilder.vi"("Errors"=w1100, "Reset Error History"=w1024) -> ("Combined Error String"=w1030:string)
    n681 = Not Equal?(x="", y=w1030) -> (x != y?=w1031:bool)
    n682 = Compound Arithmetic op=AND(w1025, w1031) -> (w1023:bool)
    n683 = case shown="True" w1023 {
      tunnel: w1030 -> [_ w1109]
      frame False {
      }
      frame True {
        n684 = call "TextToSpeech.vi"("Text To Be Spoken"=w1109) -> ()  [unwired: 9 in, 2 out]
      }
    }
    n685 = case shown="True" w1031 {
      tunnel: w1030 -> [_ w1108]
      frame False {
      }
      frame True {
        "Combined Error String" <- w1108
      }
    }
  }
  n686 = while {
    stop <- FALSE stop-if-true
    # "Set window properties"
    n687 = Not(x="Dock_Dashboard") -> (.not. x?=w1111:bool)
    n688 = First Call?() -> (First Call?: T/F=w1115:bool)
    n689 = Wait (ms)(milliseconds to wait=u32 10) -> ()  [unwired: 1 out]
    n690 = Compound Arithmetic op=OR(w1111, w1115) -> (w1113:bool)
    n691 = control-ref of="This VI"() -> (w1114:refnum<vi>)
    n692 = call "EdgeTrigger.vi"("Input Signal"=w1113) -> ("Falling Edge Trigger"=w1112:bool)  [unwired: 2 out]
    n693 = case shown="True" w1113 {
      tunnel: w1114 -> [w1120 w1127]
      tunnel: w1112 -> [w1118 _]
      frame False {
        n694 = case shown="True" w1118 {
          tunnel: T37 {"Left"=100, "Top"=100, "Right"=1390, "Bottom"=585} ("Front Panel Window:Window Bounds") -> [_ w1126]
          tunnel: w1120 -> [w1123 w1125]
          tunnel: [w1123 w1124] -> w1119
          frame False {
          }
          frame True {
            n695 = property class="VI"(reference=w1125, "Front Panel.WinBounds"=w1126) -> (reference out=w1124:refnum<vi>)  [unwired: 1 in, 1 out]
          }
        }
        n696 = property class="VI"(reference=w1119, "Front Panel.TitleBarVis"=TRUE ("Front Panel Window:Title Bar Visible")) -> ()  [unwired: 1 in, 2 out]
      }
      frame True {
        n697 = property class="VI"(reference=w1127, "Front Panel.WinBounds"=T37 {"Left"=0, "Top"=0, "Right"=1290, "Bottom"=485} ("Front Panel Window:Window Bounds"), "Front Panel.TitleBarVis"=FALSE ("Front Panel Window:Title Bar Visible")) -> ()  [unwired: 1 in, 2 out]
      }
    }
  }
